vi "Retrieve and visulize data_SE.vi"(10 "stop":bool, 11 "Field/Temperature":i32(slide) min=0 max=36 step=1) -> (0 "X line cut 2":cluster{dbl[], dbl[]}(graph), 1 "slowest":dbl=4.2894631624221803e-07, 2 "2term Intensity":dbl[][](graph), 3 "Intensity Graph":dbl[][](graph), 4 "Y line cut 2":cluster{dbl[], dbl[]}(graph)={[-1.0, -0.95, -0.9, -0.85, -0.8, -0.75, -0.7, -0.65, -0.6, -0.55, -0.5, -0.45, -0.4, -0.35, -0.3, -0.25, -0.2, -0.15, -0.1, -0.05, 0.0, 0.05, 0.1, 0.15, 0.2, 0.25, 0.3, 0.35, 0.4, 0.45, 0.5, 0.55, 0.6, 0.65, 0.7, 0.75, 0.8, 0.85, 0.9, 0.95, 1.0], [0.0, 0.0, 0.0, 0.0, 0.0, 0.0, 0.0, 0.0, 0.0, 0.0, 0.0, 0.0, 0.0, 0.0, 0.0, 0.0, 0.0, 0.0, 0.0, 0.0, 0.0, 0.0, 0.0, 0.0, 0.0, 0.0, 0.0, 0.0, 0.0, 0.0, 0.0, 0.0, 0.0, 0.0, 0.0, 0.0, 0.0, 0.0, 0.0, 0.0, 0.0]})   [LabVIEW 2016]
uses:
  <vilib>/Analysis/3filter.llb/Savitzky-Golay Filter (DBL).vi
  <vilib>/gmath/NI_Gmath.lvlib
  <vilib>/Analysis/NI_AALBase.lvlib
  <vilib>/Analysis/NI_AAL_SigProc.lvlib
panel:
  in  "Voffset - 2T":dbl format="%#_13g"
  out "Vsd vs Vsg":cluster{dbl[], dbl[]}(graph)
  out "Intensity Graph 12":dbl[][](graph)
  in  "file path (use dialog)":path=path "B:/SketchSET/SA03008H.20180718/processed/decimated_21-BG+SG_Sweep+OVERNIGHT"
  out "Scan names 2":string[](array[string])=["DSA_Vsg1", "B", "B"]
  out "Vfast index":dbl=3.0
  out "Vslow index":i32
  out "side points 4Ttemp":i32=8
  out "side points 2Ttemp":i32=12
  in  "side points 4T":i32=8
  in  "side points 2T":i32=12
  in  "Fit Points":dbl=10.0
  in  "T/B     third axis":bool
  in  "color scale":u32[](array[colorbox])=[16711680, 16772608, 6618880, 3381759, 16860, 10420479]
  in  "Voffset -2T":dbl=2e-05 format="%#_6p"
  in  "Voffset-4T":dbl=-5e-05 format="%#_4p"
  in  "Filter retrieved data?":bool=TRUE
  in  "Generate (T) or Visualize (F)":bool
  in  "Tab Control":T1(tab)=enum."3D"
  out "Comments":string="      #Vslow/#Vfast/# of IV curves/BT offset/#discarded IV curves/Manual offset:\n /101/41/1/0/0/0    \n#of fields: 1    \nField period 1 \nDecimate point 10.000000 \nScan names \nDSA_Vsg1\nB\nB \n IGOR\nX// Date: 7/19/2018 7:21 AM\nX// SA03008H\nX// \nX// Source 2 Drain 28 (lockin 1 and 7)\nX// Slow sweeping BG -5 to 5 inc. 0.1V \nX// Fast sweep SG -1 to 1 inc. 0.05V\n\nX// DSA_Vsg1=1.000000\n\nX// \nX// B= 0.000000\n\n\n\n\n\n\n\n\n\n\n\n\n\n\n\n\n\n\n\n\n\n\n\n\n\n\n\n\n\n\n\n\n\n\n\n\n\n\n\n\nX \nX Display/R 'time.SA03008H.20180718.004140'\nX AppendToGraph 'temp.SA03008H.20180718.004140'\nX AppendToGraph 'B.SA03008H.20180718.004140'\nX AppendToGraph 'Vsource.SA03008H.20180718.004140'\nX AppendToGraph 'Lockin0.SA03008H.20180718.004140'\nX AppendToGraph 'Lockin1.SA03008H.20180718.004140'\nX AppendToGraph 'Lockin2.SA03008H.20180718.004140'\nX AppendToGraph 'Lockin3.SA03008H.20180718.004140'\nX AppendToGraph 'Lockin4.SA03008H.20180718.004140'\nX AppendToGraph 'Lockin5.SA03008H.20180718.004140'\nX AppendToGraph 'B_rate.SA03008H.20180718.004140'\nX AppendToGraph 'DC0.SA03008H.20180718.004140'\nX AppendToGraph 'DC1.SA03008H.20180718.004140'\nX AppendToGraph 'DC2.SA03008H.20180718.004140'\nX AppendToGraph 'DC3.SA03008H.20180718.004140'\nX AppendToGraph 'DC4.SA03008H.20180718.004140'\nX AppendToGraph 'DC5.SA03008H.20180718.004140'\nX AppendToGraph 'DC6.SA03008H.20180718.004140'\nX AppendToGraph 'DC7.SA03008H.20180718.004140'\nX Label bottom \"x label\"\nX Label left \"y label\"\nX ModifyGraph rgb('time.SA03008H.20180718.004140')=(65280,0,0)\nX ModifyGraph rgb('temp.SA03008H.20180718.004140')=(65280,18432,0)\nX ModifyGraph rgb('B.SA03008H.20180718.004140')=(65280,36864,0)\nX ModifyGraph rgb('Vsource.SA03008H.20180718.004140')=(65280,55296,0)\nX ModifyGraph rgb('Lockin0.SA03008H.20180718.004140')=(57344,65280,0)\nX ModifyGraph rgb('Lockin1.SA03008H.20180718.004140')=(37376,65280,0)\nX ModifyGraph rgb('Lockin2.SA03008H.20180718.004140')=(18944,65280,0)\nX ModifyGraph rgb('Lockin3.SA03008H.20180718.004140')=(512,65280,0)\nX ModifyGraph rgb('Lockin4.SA03008H.20180718.004140')=(0,65280,17920)\nX ModifyGraph rgb('Lockin5.SA03008H.20180718.004140')=(0,65280,36352)\nX ModifyGraph rgb('B_rate.SA03008H.20180718.004140')=(0,65280,54784)\nX ModifyGraph rgb('DC0.SA03008H.20180718.004140')=(0,57856,65280)\nX ModifyGraph rgb('DC1.SA03008H.20180718.004140')=(0,39424,65280)\nX ModifyGraph rgb('DC2.SA03008H.20180718.004140')=(0,20992,65280)\nX ModifyGraph rgb('DC3.SA03008H.20180718.004140')=(0,2560,65280)\nX ModifyGraph rgb('DC4.SA03008H.20180718.004140')=(17408,0,65280)\nX ModifyGraph rgb('DC5.SA03008H.20180718.004140')=(35840,0,65280)\nX ModifyGraph rgb('DC6.SA03008H.20180718.004140')=(54272,0,65280)\nX ModifyGraph rgb('DC7.SA03008H.20180718.004140')=(65280,0,58368)\nX Legend/C/N=text0/J \"\\\\s('time.SA03008H.20180718.004140') time\\r\\\\s('temp.SA03008H.20180718.004140') temp\\r\\\\s('B.SA03008H.20180718.004140') B\\r\\\\s('Vsource.SA03008H.20180718.004140') Vsource\\r\\\\s('Lockin0.SA03008H.20180718.004140') Lockin0\\r\\\\s('Lockin1.SA03008H.20180718.004140') Lockin1\\r\\\\s('Lockin2.SA03008H.20180718.004140') Lockin2\\r\\\\s('Lockin3.SA03008H.20180718.004140') Lockin3\\r\\\\s('Lockin4.SA03008H.20180718.004140') Lockin4\\r\\\\s('Lockin5.SA03008H.20180718.004140') Lockin5\\r\\\\s('B_rate.SA03008H.20180718.004140') B_rate\\r\\\\s('DC0.SA03008H.20180718.004140') DC0\\r\\\\s('DC1.SA03008H.20180718.004140') DC1\\r\\\\s('DC2.SA03008H.20180718.004140') DC2\\r\\\\s('DC3.SA03008H.20180718.004140') DC3\\r\\\\s('DC4.SA03008H.20180718.004140') DC4\\r\\\\s('DC5.SA03008H.20180718.004140') DC5\\r\\\\s('DC6.SA03008H.20180718.004140') DC6\\r\\\\s('DC7.SA03008H.20180718.004140') DC7\"\nX ModifyGraph mirror(bottom)=1\nX ModifyGraph width=216\nX ModifyGraph height={Aspect,0.6}\nX ModifyGraph Log(bottom)=0\nX ModifyGraph Log(left)=0\nX \n"
  in  "Additional comments":string
  in  "Field Period":i32=1
  in  "# of fields/Temperatures":i32=1
  in  "File or Folder Path":path=path "B:/SketchSET/SA03008H.20180718/21-BG+SG_Sweep+OVERNIGHT"
  in  "Processed data folder":path=path "B:/SketchSET/SA03008H.20180718/processed"
  in  "IV file name":string="decimated_21-BG+SG_Sweep+OVERNIGHT"
  in  "IV setup":T2={"# of Vslow"=101, "# Vfast"=41, "#IV Curves at each gate"=1, "B/T offset"=0, "Discard first # curves"=0, "Manual offset"=0}
  in  "Scan names":string[](array[string])=["DSA_Vsg1", "B", "B"]
  in  "Portion of data":cluster{dbl, dbl}(slide)={1.0, 0.0} scale=0.0..1.0
  in  "Decimate point":dbl=10.0 format="%#_1f"
  in  "Extract parameters from comments?":bool=TRUE
  in  "index 2":T3={"A"=3, "B"=5, "C"=3, "D"=5, "E"=3, "N1"=2, "N2"=2, "N3"=3, "N4"=4, "A 1"=3, "A 2"=3, "C 1"=3, "C 2"=3, "E 2"=4}
  out "dV/dI 2T":cluster{dbl[], dbl[]}[](graph)
  out "dV/dI vs I":cluster{dbl[], dbl[]}[](graph)
  out "IV 2T":cluster{dbl[], dbl[]}[](graph)
  out "dI/dV 2T":cluster{dbl[], dbl[]}[](graph)
  out "dI/dV vs V":cluster{dbl[], dbl[]}[](graph)
  out "IV":cluster{dbl[], dbl[]}[](graph)
  out "IV slow 2T":cluster{dbl[], dbl[]}[](graph)
  out "dI/dV slow 2T":cluster{dbl[], dbl[]}[](graph)
  out "IV slow 4T":cluster{dbl[], dbl[]}[](graph)
  out "dI/dV slow 4T":cluster{dbl[], dbl[]}[](graph)
  out "IV vary 3rd 2T":cluster{dbl[], dbl[]}[](graph)
  out "dI/dV vary 3rd 2T":cluster{dbl[], dbl[]}[](graph)
  out "IV vary 3rd 4T":cluster{dbl[], dbl[]}[](graph)
  out "dI/dV vary 3rd 4T":cluster{dbl[], dbl[]}[](graph)
  out "Intensity Graph 2":dbl[][](graph)
  in  "X Low":dbl=-0.1 format="%#_6p"
  in  "X High":dbl=0.1 format="%#_6p"
  in  "X Step":dbl=5e-05 format="%#_6p"
  in  "Log scale?":bool
  in  "Log scale?":bool
  in  "No scale?":bool
  in  "Breakdown Low":dbl=-0.1 format="%#_6p"
  in  "Breakdown High":dbl=0.2 format="%#_6p"
  out "X scale":cluster{dbl, "X Step":dbl}={-0.09995000000000001, "X Step"=5e-05}
  out "Y scale":cluster{"Real Voltage":dbl, dbl}={"Real Voltage"=-1.0, 0.050000000000000044}
  in  "fake point value":dbl format="%#_6p"
  out "Transconductance":dbl[][](graph)
  in  "derivative bin size":dbl=15.0
  out "Field":dbl=-3.687258687258687
  out "X line cut 3":cluster{dbl[], dbl[]}(graph)
  out "X line cut 7":cluster{dbl[], dbl[]}(graph)={array[399 elements], [-0.0, -0.0, -0.0, -0.0, -0.0, -0.0, -0.0, -0.0, -0.0, -0.0, -0.0, -0.0, -0.0, -0.0, -0.0, -0.0, -0.0, -0.0, -0.0, -0.0, -0.0, -0.0, -0.0, -0.0, -0.0, -0.0, -0.0, -0.0, -0.0, -0.0, -0.0, -0.0, -0.0, -0.0, -0.0, -0.0, -0.0, -0.0, -0.0, -0.0, -0.0, -0.0, -0.0, -0.0, -0.0, -0.0, -0.0, -0.0, -0.0, -0.0, -0.0, -0.0, -0.0, -0.0, -0.0, -0.0, -0.0, -0.0, -0.0, -0.0, -0.0, -0.0, -0.0, -0.0, -0.0, -0.0, -0.0, -0.0, -0.0, -0.0, -0.0, -0.0, -0.0, -0.0, -0.0, -0.0, -0.0, -0.0, -0.0, -0.0, -0.0, -0.0, -0.0, -0.0, -0.0, -0.0, -0.0, -0.0, -0.0, -0.0, -0.0, -0.0, -0.0, -0.0, -0.0, -0.0, -0.0, -0.0, -0.0, -0.0, -0.0, -0.0, -0.0, -0.0, -0.0, -0.0, -0.0, -0.0, -0.0, -0.0, -0.0, -0.0, -0.0, -0.0, -0.0, -0.0, -0.0, -0.0, -0.0, -0.0, -0.0, -0.0, -0.0, -0.0, -0.0, -0.0, -0.0, -0.0, -0.0, -0.0, -0.0, -0.0, -0.0, -0.0, -0.0, -0.0, -0.0, -0.0, -0.0, -0.0, -0.0, -0.0, -0.0, -0.0, -0.0, -0.0, -0.0, -0.0, -0.0, -0.0, -0.0, -0.0, -0.0, -0.0, -0.0, -0.0, -0.0, -0.0, -0.0, -0.0, -0.0, -0.0, -0.0, -0.0, -0.0, -0.0, -0.0, -0.0, -0.0, -0.0, -0.0, -0.0, -0.0, -0.0, -0.0, -0.0, -0.0, -0.0, -0.0, -0.0, -0.0, -0.0, -0.0, -0.0, -0.0, -0.0, -0.0, -0.0, -0.0, -0.0, -0.0, -0.0, -0.0, -0.0, -0.0, -0.0, -0.0, -0.0, -0.0, -0.0, -0.0, -0.0, -0.0, -0.0, -0.0, -0.0, -0.0, -0.0, -0.0, -0.0, -0.0, -0.0, -0.0, -0.0, -0.0, -0.0, -0.0, -0.0, -0.0, -0.0, -0.0, -0.0, -0.0, -0.0, -0.0, -0.0, -0.0, -0.0, -0.0, -0.0, -0.0, -0.0, -0.0, -0.0, -0.0, -0.0, -0.0, -0.0, -0.0, -0.0, -0.0, -0.0, -0.0, -0.0, -0.0, -0.0, -0.0, -0.0, -0.0, -0.0, -0.0, -0.0, -0.0, -0.0, -0.0, -0.0, -0.0, -0.0, -0.0, -0.0, -0.0, -0.0, -0.0, -0.0, -0.0, -0.0, -0.0, -0.0, -0.0, -0.0, -0.0, -0.0, -0.0, -0.0, -0.0, -0.0, -0.0, -0.0, -0.0, -0.0, -0.0, -0.0, -0.0, -0.0, -0.0, -0.0, -0.0, -0.0, -0.0, -0.0, -0.0, -0.0, -0.0, -0.0, -0.0, -0.0, -0.0, -0.0, -0.0, -0.0, -0.0, -0.0, -0.0, -0.0, -0.0, -0.0, -0.0, -0.0, -0.0, -0.0, -0.0, -0.0, -0.0, -0.0, -0.0, -0.0, -0.0, -0.0, -0.0, -0.0, -0.0, -0.0, -0.0, -0.0, -0.0, -0.0, -0.0, -0.0, -0.0, -0.0, -0.0, -0.0, -0.0, -0.0, -0.0, -0.0, -0.0, -0.0, -0.0, -0.0, -0.0, -0.0, -0.0, -0.0, -0.0, -0.0, -0.0, -0.0, -0.0, -0.0, -0.0, -0.0, -0.0, -0.0, -0.0, -0.0, -0.0, -0.0, -0.0, -0.0, -0.0, -0.0, -0.0, -0.0, -0.0, -0.0, -0.0, -0.0, -0.0, -0.0, -0.0, -0.0, -0.0, -0.0, -0.0, -0.0, -0.0, -0.0, -0.0, -0.0, -0.0, -0.0, -0.0, -0.0, -0.0, -0.0, -0.0, -0.0, -0.0, -0.0, -0.0, -0.0, -0.0, -0.0, -0.0, -0.0, -0.0, -0.0, -0.0]}
  out "Y line cut 8":cluster{dbl[], dbl[]}(graph)={[-1.0, -0.95, -0.9, -0.85, -0.8, -0.75, -0.7, -0.65, -0.6, -0.55, -0.5, -0.45, -0.4, -0.35, -0.3, -0.25, -0.2, -0.15, -0.1, -0.05, 0.0, 0.05, 0.1, 0.15, 0.2, 0.25, 0.3, 0.35, 0.4, 0.45, 0.5, 0.55, 0.6, 0.65, 0.7, 0.75, 0.8, 0.85, 0.9, 0.95, 1.0], [-0.0, -0.0, -0.0, -0.0, -0.0, -0.0, -0.0, -0.0, -0.0, -0.0, -0.0, -0.0, -0.0, -0.0, -0.0, -0.0, -0.0, -0.0, -0.0, -0.0, -0.0, -0.0, -0.0, -0.0, -0.0, -0.0, -0.0]}
  out "Y line cut":cluster{"Vfast":dbl[], dbl[]}(graph)
  out "X line cut":cluster{dbl[], dbl[]}(graph)
  out "2 term trans":dbl[][](graph)
  in  "X Step 2T":dbl=4e-05 format="%#_6p"
  in  "X High 2T":dbl=0.1 format="%#_6p"
  in  "X Low 2T":dbl=-0.1 format="%#_6p"
  in  "Log scale?":bool
  in  "Log scale?":bool
  in  "fake point value 2":dbl format="%#_6p"
  out "2term trans X line cut":cluster{dbl[], dbl[]}(graph)
  out "2term trans Y line cut":cluster{"Vfast":dbl[], dbl[]}(graph)
  in  "e^2/h?":bool
  out "2term Intensity Current vs. Voltage":dbl[][](graph)
  in  "width X 6":dbl=1e-09 min=1.0 format="%#_6p"
  in  "width Y 6":dbl=1e-09 min=1.0 format="%#_6p"
  out "Y line cut 6":cluster{"Vfast":dbl[], dbl[]}(graph)={"Vfast"=[-5.0, -4.9, -4.8, -4.7, -4.6, -4.5, -4.4, -4.3, -4.2, -4.1, -4.0, -3.9, -3.8, -3.7, -3.5999999999999996, -3.5, -3.4, -3.3, -3.2, -3.0999999999999996, -3.0, -2.9, -2.8, -2.6999999999999997, -2.5999999999999996, -2.5, -2.4, -2.3, -2.1999999999999997, -2.0999999999999996, -2.0, -1.9, -1.7999999999999998, -1.6999999999999997, -1.5999999999999996, -1.5, -1.4, -1.2999999999999998, -1.1999999999999997, -1.0999999999999996, -1.0, -0.8999999999999995, -0.7999999999999998, -0.7000000000000002, -0.5999999999999996, -0.5, -0.39999999999999947, -0.2999999999999998, -0.1999999999999993, -0.09999999999999964, 0.0, 0.10000000000000053, 0.20000000000000018, 0.3000000000000007, 0.40000000000000036, 0.5, 0.6000000000000005, 0.7000000000000002, 0.8000000000000007, 0.9000000000000004, 1.0, 1.1000000000000005, 1.2000000000000002, 1.3000000000000007, 1.4000000000000004, 1.5, 1.6000000000000005, 1.7000000000000002, 1.8000000000000007, 1.9000000000000004, 2.0, 2.1000000000000005, 2.2, 2.3000000000000007, 2.4000000000000004, 2.5, 2.6000000000000005, 2.7, 2.8000000000000007, 2.9000000000000004, 3.0, 3.0999999999999996, 3.200000000000001, 3.3000000000000007, 3.4000000000000004, 3.5, 3.5999999999999996, 3.700000000000001, 3.8000000000000007, 3.9000000000000004, 4.0, 4.1, 4.200000000000001, 4.300000000000001, 4.4, 4.5, 4.600000000000001, 4.700000000000001, 4.800000000000001, 4.9, 5.0], [0.02727272727272727, 0.02727272727272727, 0.02727272727272727, 0.02727272727272727, 0.02727272727272727, 0.02727272727272727, 0.02727272727272727, 0.02727272727272727, 0.02727272727272727, 0.02727272727272727, 0.02727272727272727, 0.02727272727272727, 0.02727272727272727, 0.02727272727272727, 0.02727272727272727, 0.02727272727272727, 0.02727272727272727, 0.02727272727272727, 0.02727272727272727, 0.02727272727272727, 0.02727272727272727, 0.02727272727272727, 0.02727272727272727, 0.02727272727272727, 0.02727272727272727, 0.02727272727272727, 0.02727272727272727, 0.02727272727272727, 0.02727272727272727, 0.02727272727272727, 0.02727272727272727, 0.02727272727272727, 0.02727272727272727, 0.02727272727272727, 0.02727272727272727, 0.02727272727272727, 0.02727272727272727, 0.02727272727272727, 0.02727272727272727, 0.02727272727272727, 0.02727272727272727, 0.02727272727272727, 0.02727272727272727, 0.02727272727272727, 0.02727272727272727, 0.02727272727272727, 0.02727272727272727, 0.02727272727272727, 0.02727272727272727, 0.02727272727272727, 0.02727272727272727, 0.02727272727272727, 0.02727272727272727, 0.02727272727272727, 0.02727272727272727, 0.02727272727272727, 0.02727272727272727, 0.02727272727272727, 0.02727272727272727, 0.02727272727272727, 0.02727272727272727, 0.02727272727272727, 0.02727272727272727, 0.02727272727272727, 0.02727272727272727, 0.02727272727272727, 0.02727272727272727, 0.02727272727272727, 0.02727272727272727, 0.02727272727272727, 0.02727272727272727, 0.02727272727272727, 0.02727272727272727, 0.02727272727272727, 0.02727272727272727, 0.02727272727272727, 0.02727272727272727, 0.02727272727272727, 0.02727272727272727, 0.02727272727272727, 0.02727272727272727, 0.02727272727272727, 0.02727272727272727, 0.02727272727272727, 0.02727272727272727, 0.02727272727272727, 0.02727272727272727, 0.02727272727272727, 0.02727272727272727, 0.02727272727272727, 0.02727272727272727, 0.02727272727272727, 0.02727272727272727, 0.02727272727272727, 0.02727272727272727, 0.02727272727272727, 0.02727272727272727, 0.02727272727272727, 0.02727272727272727, 0.02727272727272727, 0.02727272727272727]}
  out "X line cut 6":cluster{dbl[], dbl[]}(graph)
  out "Y line cut 5":cluster{"Vfast":dbl[], dbl[]}(graph)={"Vfast"=[-1.0, -0.95, -0.9, -0.85, -0.8, -0.75, -0.7, -0.65, -0.6, -0.55, -0.5, -0.45, -0.4, -0.35, -0.3, -0.25, -0.2, -0.15, -0.1, -0.05, 0.0, 0.05, 0.1, 0.15, 0.2, 0.25, 0.3, 0.35, 0.4, 0.45, 0.5, 0.55, 0.6, 0.65, 0.7, 0.75, 0.8, 0.85, 0.9, 0.95, 1.0], [0.049999999999999996, 0.049999999999999996, 0.049999999999999996, 0.049999999999999996, 0.049999999999999996, 0.049999999999999996, 0.049999999999999996, 0.049999999999999996, 0.049999999999999996, 0.049999999999999996, 0.049999999999999996, 0.049999999999999996, 0.049999999999999996, 0.049999999999999996, 0.049999999999999996, 0.049999999999999996, 0.049999999999999996, 0.049999999999999996, 0.049999999999999996, 0.049999999999999996, 0.049999999999999996, 0.049999999999999996, 0.049999999999999996, 0.049999999999999996, 0.049999999999999996, 0.049999999999999996, 0.049999999999999996, 0.049999999999999996, 0.049999999999999996, 0.049999999999999996, 0.049999999999999996, 0.049999999999999996, 0.049999999999999996, 0.049999999999999996, 0.049999999999999996, 0.049999999999999996, 0.049999999999999996, 0.049999999999999996, 0.049999999999999996, 0.049999999999999996, 0.049999999999999996]}
  out "X line cut 5":cluster{dbl[], dbl[]}(graph)
  out "Intensity Graph 6":dbl[][](graph)
  in  "X Step 4t":dbl=1e-10 format="%#_6p"
  in  "X High 4t":dbl=3e-08 format="%#_6p"
  in  "X Low 4t":dbl=-3e-08 format="%#_6p"
  in  "Log scale? 3":bool
  in  "Log scale? 2":bool
  out "Intensity Graph 5":dbl[][](graph)
  in  "fake point value 3":dbl=0.05 format="%#_6p"
  in  "width X 5":dbl=1e-09 min=1.0 format="%#_6p"
  in  "width Y 5":dbl=1e-09 min=1.0 format="%#_6p"
  out "Y line cut 4":cluster{"Vfast":dbl[], dbl[]}(graph)
  out "X line cut 4":cluster{dbl[], dbl[]}(graph)
  out "Intensity Graph 8":dbl[][](graph)
  in  "X Step 2t":dbl=1e-11 format="%#_6p"
  in  "X High 2t":dbl=1e-09 format="%#_6p"
  in  "X Low 2t":dbl=-2e-09 format="%#_6p"
  in  "Log scale? 5":bool
  in  "Log scale? 4":bool
  out "Intensity Graph 7":dbl[][](graph)
  in  "fake pt value 4":dbl=0.05 format="%#_6p"
  out "Intensity Graph 11":dbl[][](graph)
  out "Intensity Graph 10":dbl[][](graph)
  out "Intensity Graph 9":dbl[][](graph)
  out "Transconductance 2":dbl[][](graph)
  in  "derivative bin size 2":dbl=10.0
  in  "width":i32=3 min=3
  in  "threshold":dbl format="%0.2f"
  out "vertical peak diff":dbl[](array[numeric])
  out "Array 2":dbl[](array[numeric])
  out "Y line cut 9":cluster{dbl[], dbl[]}[](graph)
  in  "width 2":i32=3 min=3
  in  "threshold 2":dbl format="%0.2f"
  in  "calc alpha?":bool
  out "XY Graph":cluster{dbl[], dbl[]}(graph)
  # "I+"
  # "V+"
  # "Vsg1"
  # "Vsgw"
  # "Vsg2"
  # "V-"
  # "I-"
  # "Output"
  # "Vfast"
  # "Vslow"
  # "Vslowest"
  # "Vfast"
  # "Vslow"
  # "Vslowest"
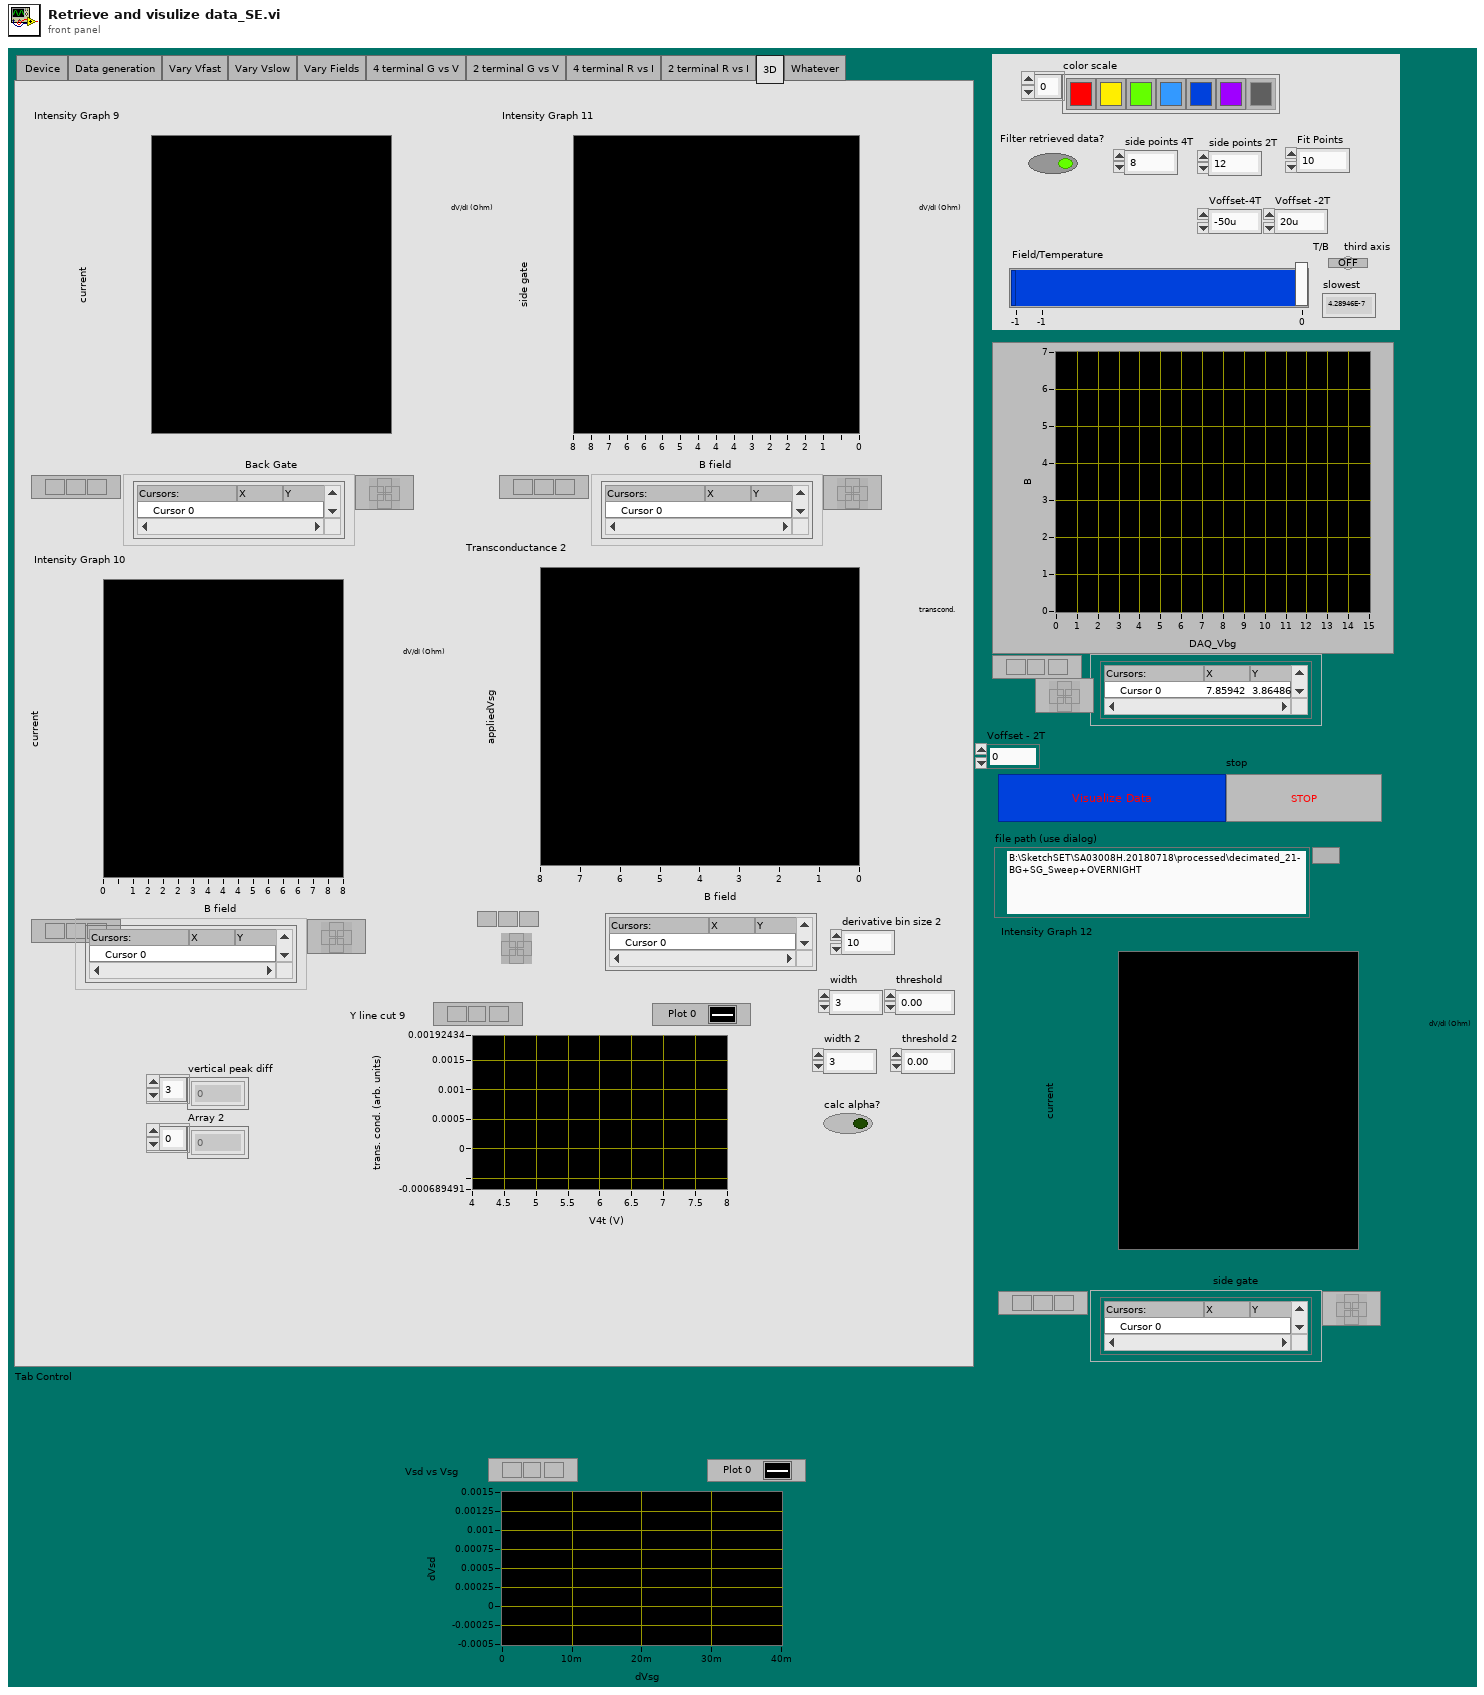
[diagram p1: front panel]
types:
  T1 = enum32{"Device ", "Data generation", "Vary Vfast", "Vary Vslow", "Vary Fields", "4 terminal G vs V", "2 terminal G vs V", "4 terminal R vs I", "2 terminal R vs I", "3D", "Whatever"}
  T2 = cluster{"# of Vslow":i32, "# Vfast":i32, "#IV Curves at each gate":i32, "B/T offset":i32, "Discard first # curves":i32, "Manual offset":i32}
  T3 = cluster{"A":i32, "B":i32, "C":i32, "D":i32, "E":i32, "N1":i32, "N2":i32, "N3":i32, "N4":i32, "A 1":i32, "A 2":i32, "C 1":i32, "C 2":i32, "E 2":i32}
  T4 = enum16{"open", "replace", "create", "open or create", "replace or create", "replace or create with confirmation"}
  T5 = cluster{"IV":cluster{dbl[], dbl[]}[][][], "IV-2T":cluster{dbl[], dbl[]}[][][], "Vfast":dbl[][], "Vslow":dbl[], "Vslowest":dbl[], "Comments":string, "Scan names":string[]}[]
  T6 = cluster{"IV":cluster{dbl[], dbl[]}[][][], "IV-2T":cluster{dbl[], dbl[]}[][][], "Vfast":dbl[][], "Vslow":dbl[], "Vslowest":dbl[], "Comments":string, "Scan names":string[]}
  T7 = cluster{"Decimated Array":dbl[], "Decimated Array":dbl[]}
  T8 = cluster{"Decimated Array":dbl[], "Decimated Array":dbl[]}[][][]
  T9 = cluster{"Decimated Array":dbl[], "Filtered X":dbl[]}
  T10 = cluster{"Decimated Array":dbl[], "Decimated Array":dbl[]}[][]
  T11 = cluster{"Decimated Array":dbl[], "Decimated Array":dbl[]}[]
  T12 = cluster{"X Low 2T":dbl, "X High 2T":dbl, "X Step 2T":dbl, "Voffset -2T":dbl}
  T13 = cluster{"Decimated X values":dbl[], "Transconductance":dbl[]}
  T14 = cluster{"X Low 2t":dbl, "X High 2t":dbl, "X Step 2t":dbl, "Voffset - 2T":dbl}
  T15 = cluster{"IV":cluster{dbl[], dbl[]}[][][], "IV-2T":cluster{dbl[], dbl[]}[][][], "Vfast":dbl[][], "Vslow":dbl[], dbl[], string, "Scan names":string[]}
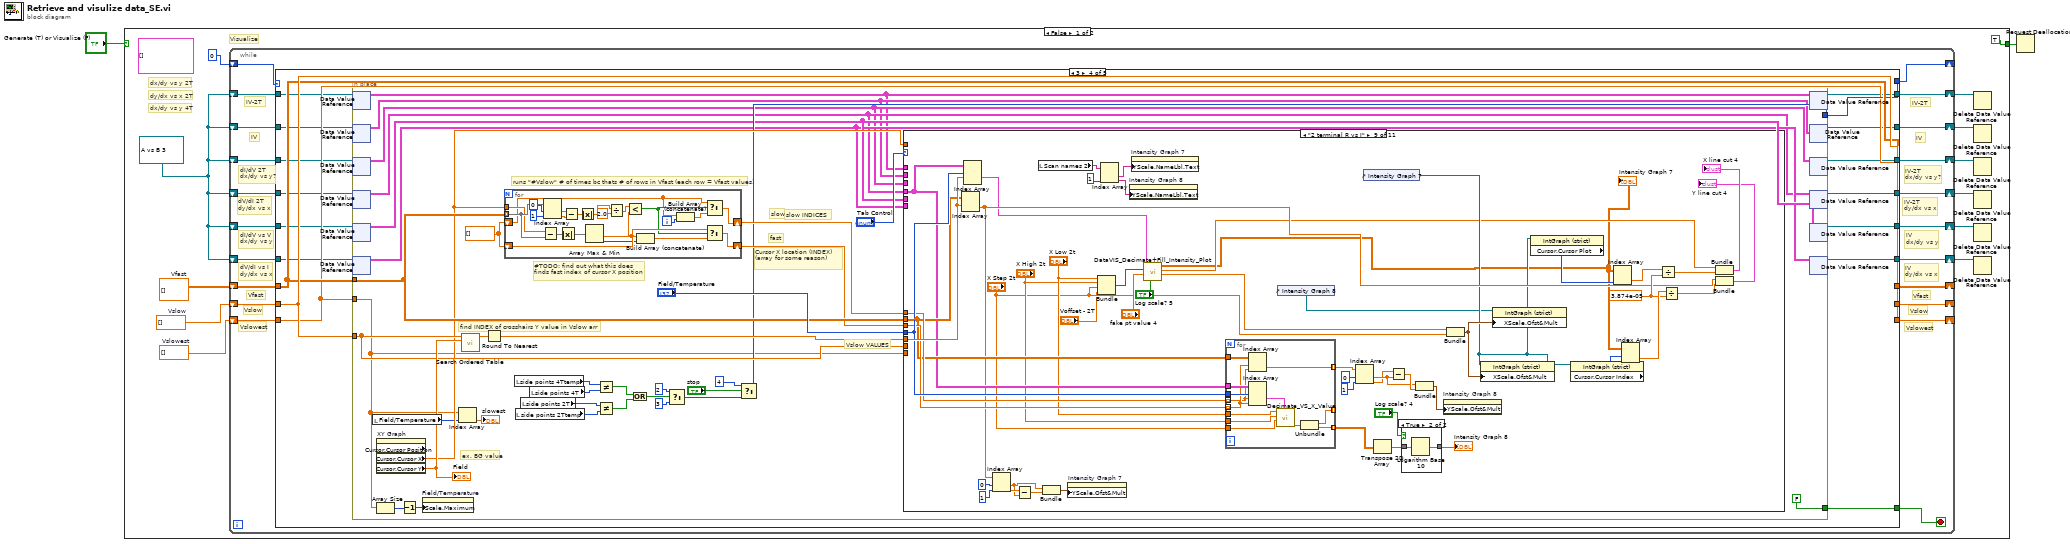
[diagram p0: block diagram]
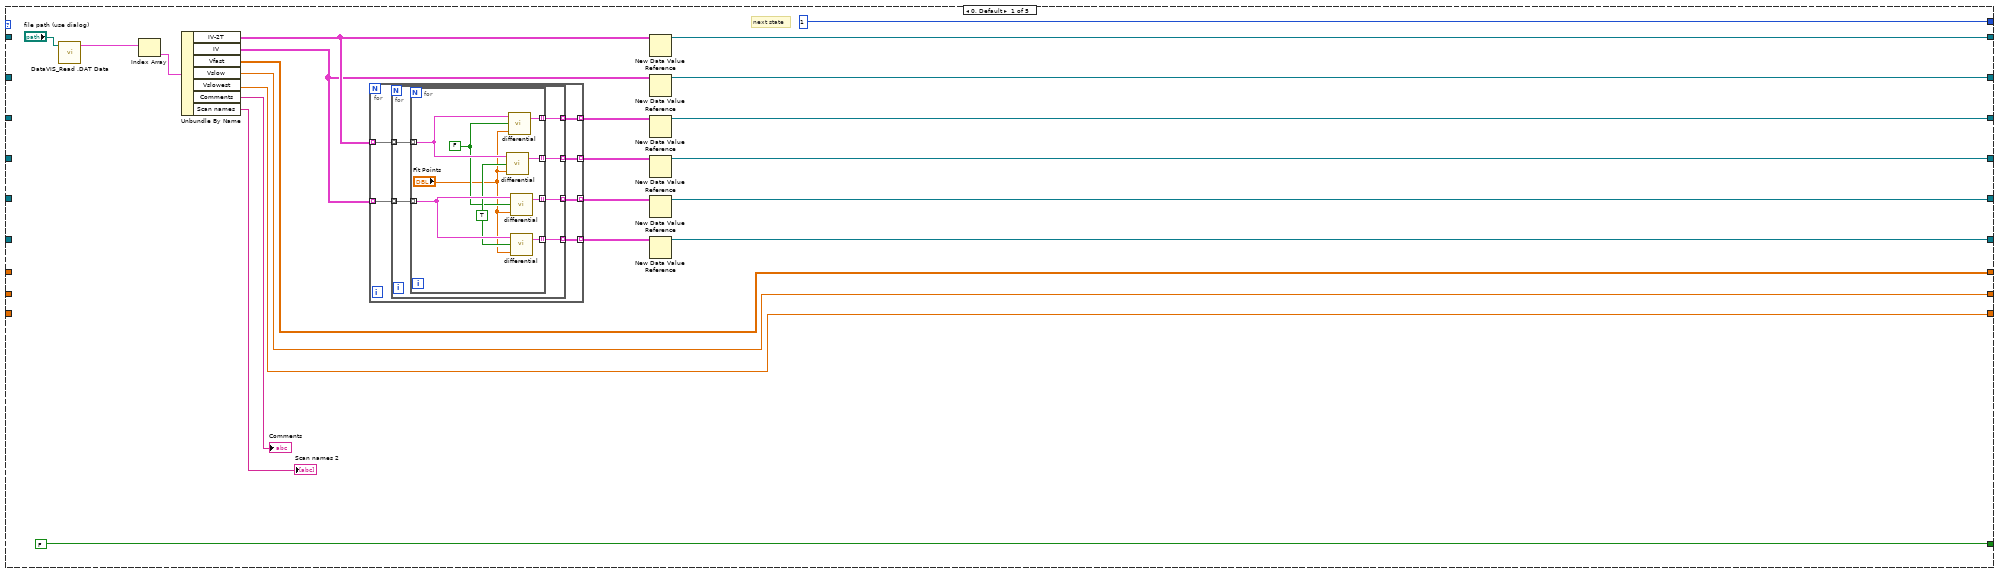
[diagram p2: hidden frame]
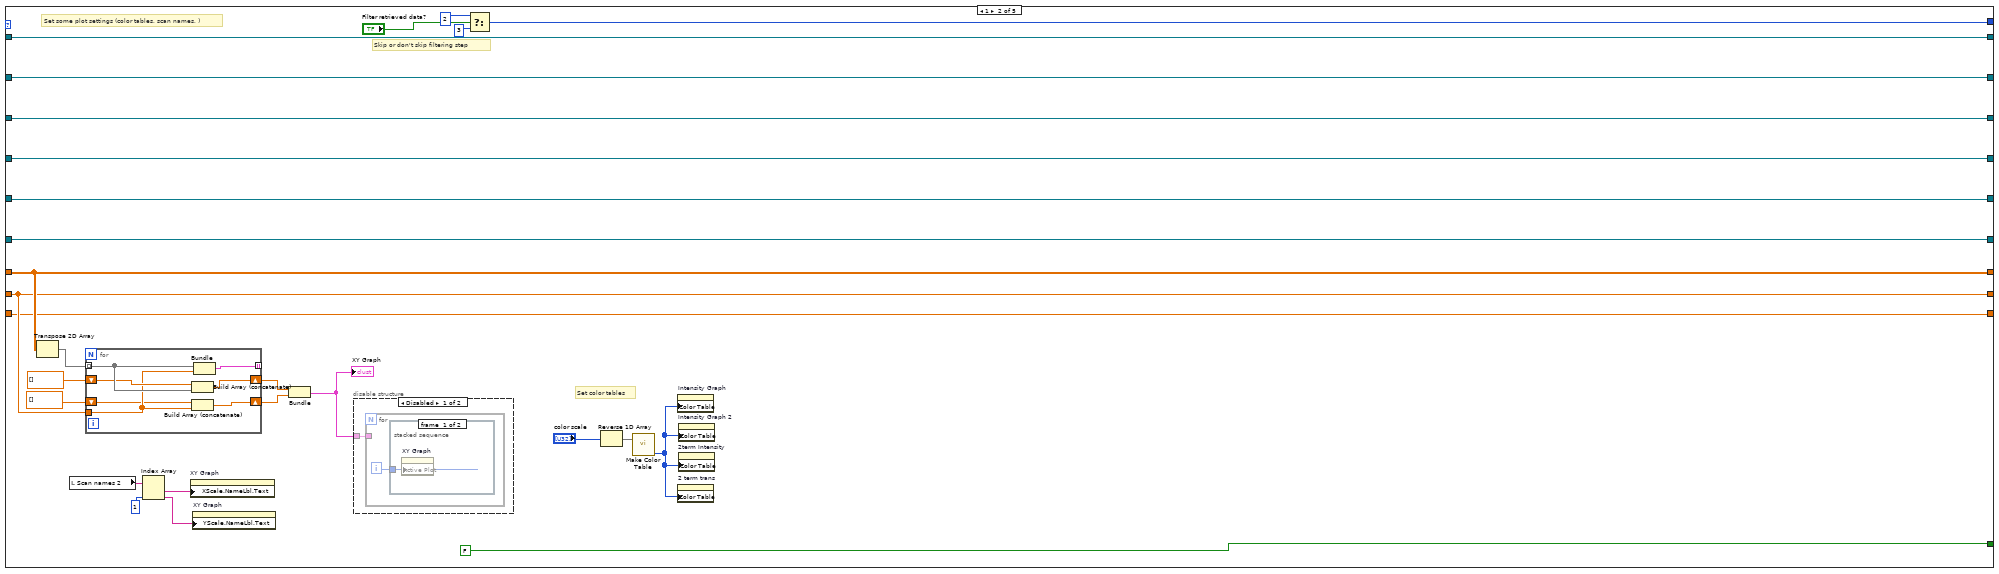
[diagram p3: hidden frame]
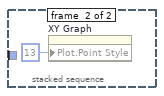
[diagram p4: hidden frame]
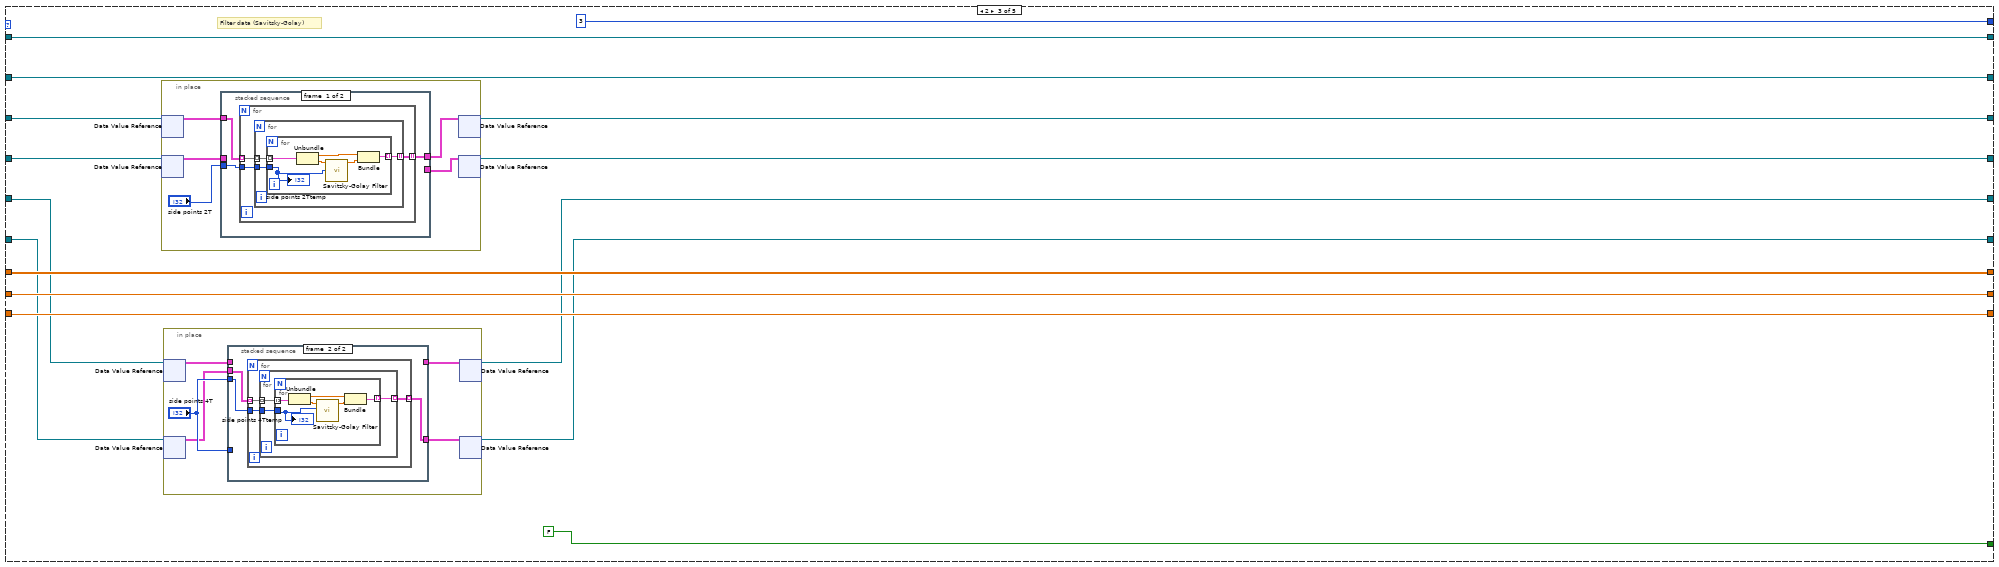
[diagram p6: hidden frame]
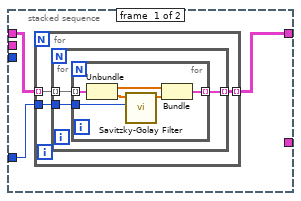
[diagram p7: hidden frame]
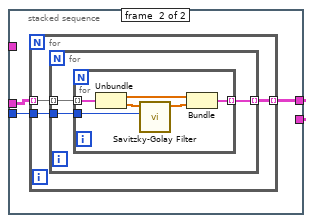
[diagram p8: hidden frame]
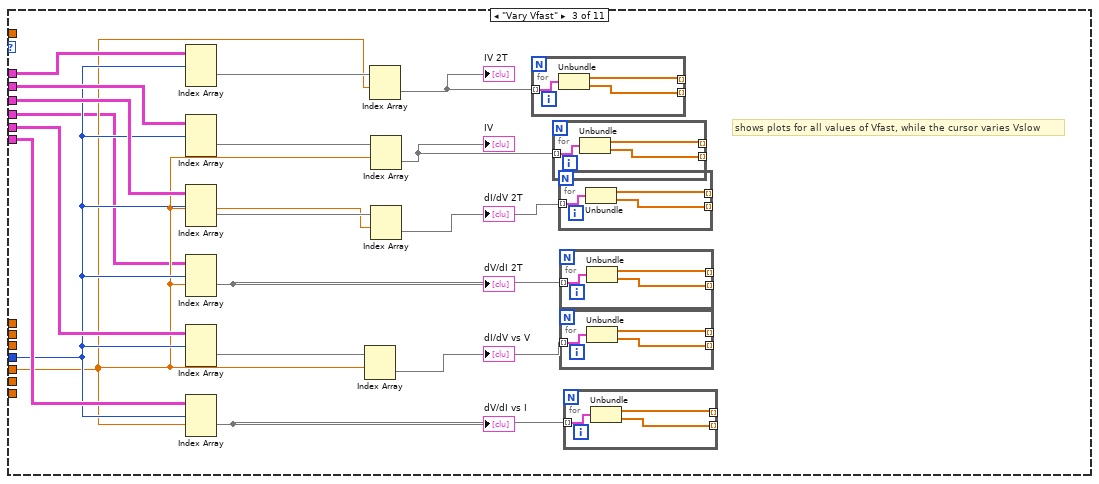
[diagram p11: hidden frame]
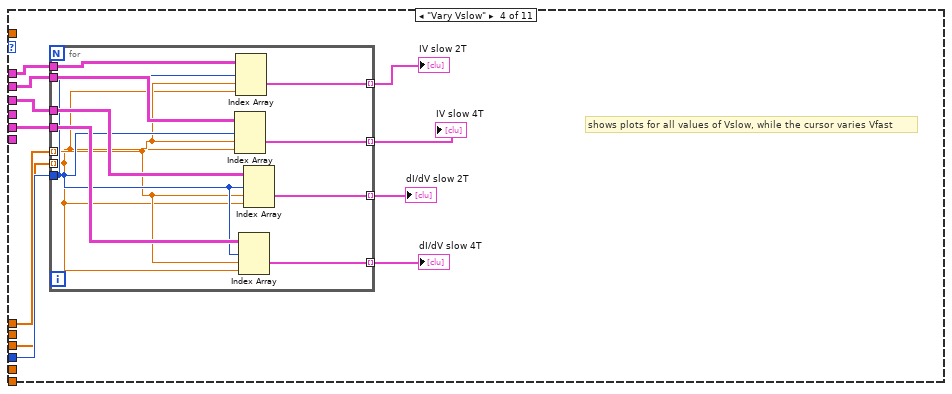
[diagram p12: hidden frame]
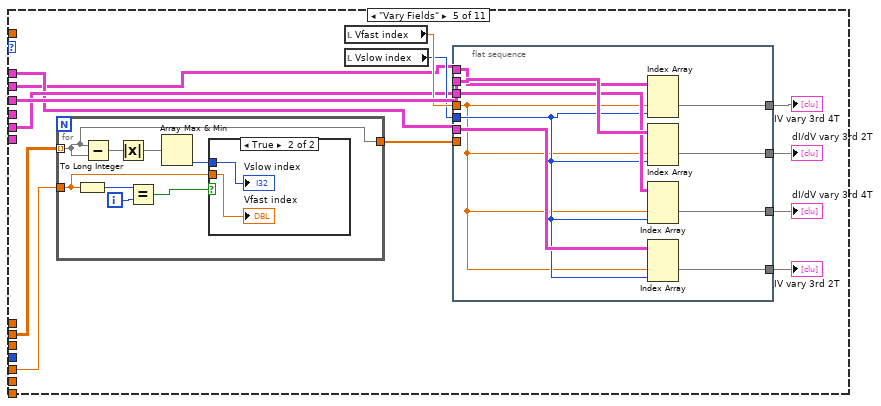
[diagram p13: hidden frame]
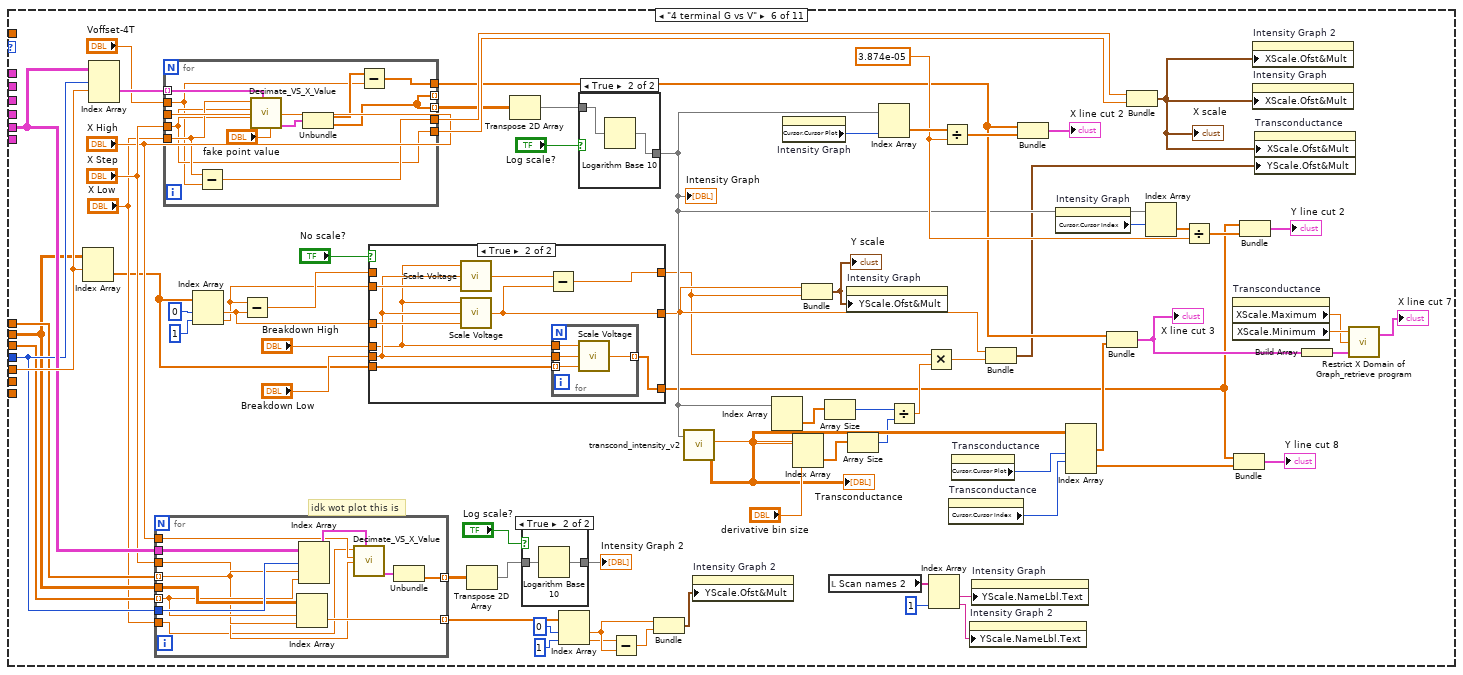
[diagram p15: hidden frame]
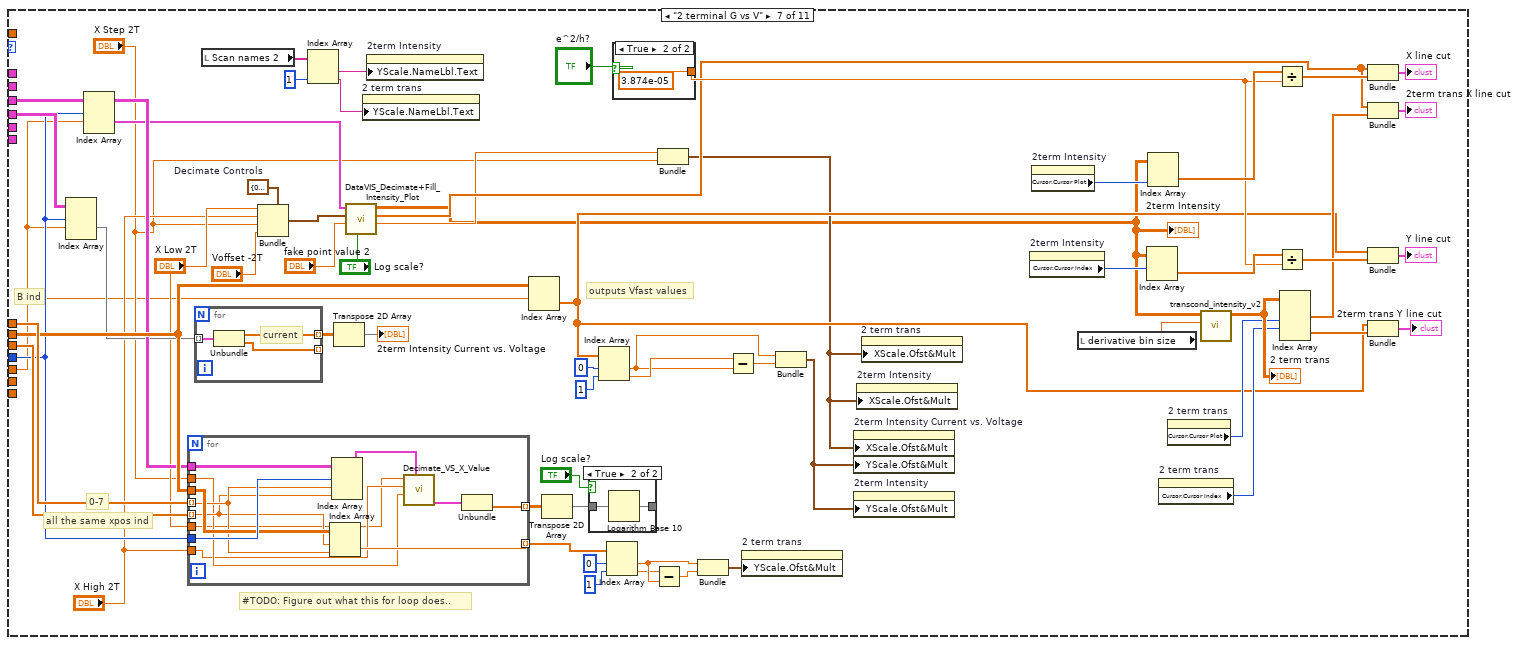
[diagram p19: hidden frame]
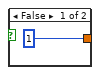
[diagram p20: hidden frame]
diagram:
  n1 = case shown="False" "Generate (T) or Visualize (F)" {
    tunnel: [TRUE TRUE] -> w1
    frame False {
      w3 = dbl[] []  # Vslowest
      w11 = refnum<data-value> refnum ("data value reference")
      w13 = dbl[] []  # Vslow
      w14 = dbl[][] []  # Vfast
      (unwired) cluster{dbl[], dbl[]}[][][] [] ("IV")
      # "Visualize"
      # "dx/dy vs y 4T"
      # "dy/dx vs x 2T"
      # "dx/dy vs y 2T"
      n2 = while {
        shift-right: [w31] -> _
        shift-left: 0 -> [w35]
        shift-right: [w15] -> w10
        shift-left: w11 -> [w16]
        shift-right: [w26] -> w9
        shift-left: w11 -> [w21]
        shift-right: [w25] -> w8
        shift-left: w11 -> [w20]
        shift-right: [w24] -> w7
        shift-left: w11 -> [w19]
        shift-right: [w23] -> w6
        shift-left: w11 -> [w18]
        shift-right: [w22] -> w5
        shift-left: w11 -> [w17]
        shift-right: [w34] -> _
        shift-left: w14 -> [w30]
        shift-right: [w33] -> _
        shift-left: w13 -> [w29]
        shift-right: [w32] -> _
        shift-left: w3 -> [w28]
        stop <- w27 stop-if-true
        # "dI/dV vs V\ndx/dy vs y"
        # "dV/dI vs I\ndy/dx vs x"
        # "dV/dI 2T\ndy/dx vs x"
        # "dI/dV 2T\ndx/dy vs y?"
        # "IV"
        # "IV-2T"
        # "Vfast"
        # "Vslowest"
        # "Vslow"
        # "IV\ndx/dy vs y"
        # "IV\ndy/dx vs x"
        # "IV-2T\ndy/dx vs x"
        # "IV-2T\ndx/dy vs y?"
        # "IV"
        # "IV-2T"
        # "Vfast"
        # "Vslowest"
        # "Vslow"
        n3 = case shown="3" w35 {
          tunnel: [w54 w104 w122 w206 w848] -> w26
          tunnel: [w52 w103 w118 w204 w846] -> w24
          tunnel: [w51 w98 w131 w203 w845] -> w23
          tunnel: [w50 w99 w130 w202 w844] -> w22
          tunnel: [w37 w102 w128 w217 w850] -> w34
          tunnel: [w36 w101 w127 w218 w854] -> w33
          tunnel: [w57 w100 w126 w214 w853] -> w32
          tunnel: w16 -> [_ w79 w124 w213 w849]
          tunnel: w20 -> [_ w80 w121 w210 w847]
          tunnel: w21 -> [_ w104 w123 w211 w848]
          tunnel: w19 -> [_ w103 w120 w209 w846]
          tunnel: w18 -> [_ w98 w131 w208 w845]
          tunnel: w17 -> [_ w99 w130 w207 w844]
          tunnel: [1 w91 3 w216 4] -> w31
          tunnel: w30 -> [_ w102 w128 w217 w850]
          tunnel: w29 -> [_ w101 w127 w218 w854]
          tunnel: w28 -> [_ w100 w126 w214 w853]
          tunnel: [FALSE FALSE FALSE w215 TRUE] -> w27
          tunnel: [w53 w80 w119 w205 w847] -> w25
          tunnel: [w49 w79 w117 w212 w849] -> w15
          frame 0, Default {
            # "next state"
            n4 = call "DataVIS_Read .DAT Data.vi"("file path (use dialog)"="file path (use dialog)") -> ("Array"=w48:T5)  [unwired: 9 in, 1 out]
            n5 = Index Array(array=w48) -> (element=w47:T6)  [unwired: 1 in]
            n6 = Unbundle By Name(w47) -> ("IV-2T"=w39:cluster{dbl[], dbl[]}[][][], "IV"=w38:cluster{dbl[], dbl[]}[][][], "Vfast"=w37:dbl[][], "Vslow"=w36:dbl[], "Vslowest"=w57:dbl[], "Comments"=→"Comments":string, "Scan names"=→"Scan names 2":string[])
            n7 = for {
              tunnel: w38 -> [w63] mode=indexing
              tunnel: [w62] -> w40 mode=indexing
              tunnel: [w61] -> w41 mode=indexing
              tunnel: w39 -> [w60] mode=indexing
              tunnel: [w59] -> w42 mode=indexing
              tunnel: [w58] -> w43 mode=indexing
              n8 = for {
                tunnel: w63 -> [w69] mode=indexing
                tunnel: [w68] -> w62 mode=indexing
                tunnel: [w67] -> w61 mode=indexing
                tunnel: w60 -> [w66] mode=indexing
                tunnel: [w65] -> w59 mode=indexing
                tunnel: [w64] -> w58 mode=indexing
                n9 = for {
                  tunnel: w69 -> [w77] mode=indexing
                  tunnel: [w78] -> w68 mode=indexing
                  tunnel: [w75] -> w67 mode=indexing
                  tunnel: w66 -> [w74] mode=indexing
                  tunnel: [w71] -> w65 mode=indexing
                  tunnel: [w70] -> w64 mode=indexing
                  w73 = FALSE ("dy/dx vs x")
                  w76 = TRUE ("dy/dx vs x")
                  n10 = call <userlib>:"differential.vi"("Numeric"="Fit Points", "dy/dx vs x"=w76, "A vs B 2"=w74) -> ("A vs B 3"=w71:T7)  [unwired: 1 in]
                  n11 = call <userlib>:"differential.vi"("Numeric"="Fit Points", "dy/dx vs x"=w73, "A vs B 2"=w74) -> ("A vs B 3"=w70:T7)  [unwired: 1 in]
                  n12 = call <userlib>:"differential.vi"("Numeric"="Fit Points", "dy/dx vs x"=w73, "A vs B 2"=w77) -> ("A vs B 3"=w75:T7)  [unwired: 1 in]
                  n13 = call <userlib>:"differential.vi"("Numeric"="Fit Points", "dy/dx vs x"=w76, "A vs B 2"=w77) -> ("A vs B 3"=w78:T7)  [unwired: 1 in]
                }
              }
            }
            n14 = New Data Value Reference(data value=w39) -> (data value reference=w51:refnum<data-value>)  [unwired: 1 in, 1 out]
            n15 = New Data Value Reference(data value=w38) -> (data value reference=w50:refnum<data-value>)  [unwired: 1 in, 1 out]
            n16 = New Data Value Reference(data value=w43) -> (data value reference=w49:refnum<data-value>)  [unwired: 1 in, 1 out]
            n17 = New Data Value Reference(data value=w42) -> (data value reference=w54:refnum<data-value>)  [unwired: 1 in, 1 out]
            n18 = New Data Value Reference(data value=w41) -> (data value reference=w53:refnum<data-value>)  [unwired: 1 in, 1 out]
            n19 = New Data Value Reference(data value=w40) -> (data value reference=w52:refnum<data-value>)  [unwired: 1 in, 1 out]
          }
          frame 1 {
            # "Set some plot settings (color tables, scan names, )"
            # "Skip or don't skip filtering step"
            # "Set color tables"
            n20 = Transpose 2D Array(2D array=w102) -> (transposed array=w105:dbl[][])
            n21 = local read "Scan names 2"() -> (w89:string[])
            n22 = for {
              tunnel: w105 -> [w115] mode=indexing
              tunnel: [w116] -> _ mode=indexing
              tunnel: w101 -> [w112]
              shift-right: [w113] -> w83
              shift-left: dbl[] [] -> [w114]
              shift-right: [w111] -> w82
              shift-left: dbl[] [] -> [w110]
              n23 = Build Array (concatenate)(w114, w115) -> (w113:dbl[])
              n24 = Build Array (concatenate)(w110, w112) -> (w111:dbl[])
              n25 = Bundle(w115, "Vslow"=w112) -> (w116:cluster{dbl[], "Vslow":dbl[]})  [unwired: 1 in]
            }
            n26 = Index Array(array=w89, index #2=1 ("index")) -> (element #1=w87:string, element #2=w86:string)  [unwired: 1 in]
            n27 = property on="XY Graph" class="XYGraph (strict)"("XScale.NameLbl.Text"=w87) -> ()  [unwired: 2 in, 2 out]
            n28 = property on="XY Graph" class="XYGraph (strict)"("YScale.NameLbl.Text"=w86) -> ()  [unwired: 2 in, 2 out]
            n29 = Bundle(w83, w82) -> (w81:cluster{dbl[], dbl[]})  [unwired: 1 in]
            "XY Graph" <- w81
            n30 = disable-structure shown="Disabled" {
              disable-tunnel: w81 -> [w106 _]
              frame Disabled {
                n31 = for {
                  tunnel: w106 -> [_]
                  i -> [w107]
                  n32 = stacked-sequence {
                    tunnel: w107 -> [w108 _]
                    frame #0 {
                      n33 = property on="XY Graph" class="XYGraph (strict)"("Active Plot"=w108) -> ()  [unwired: 2 in, 2 out]
                    }
                    frame #1 {
                      n34 = property on="XY Graph" class="XYGraph (strict)"("Plot.Point Style"=u8 13) -> ()  [unwired: 2 in, 2 out]
                    }
                  }
                }
              }
              frame Enabled {
              }
            }
            n35 = Select(t=2, s="Filter retrieved data?", f=3) -> (s? t:f=w91:i32)
            n36 = Reverse 1D Array(array="color scale") -> (reversed array=w96:u32[])
            n37 = call <userlib>:"Make Color Table.vi"("Array"=w96) -> ("Color Tbl"=w95:u32[])  [unwired: 1 in, 3 out]
            n38 = property on="Intensity Graph" class="IntGraph (strict)"("Color Table"=w95) -> ()  [unwired: 2 in, 2 out]
            n39 = property on="2 term trans" class="IntGraph (strict)"("Color Table"=w95) -> ()  [unwired: 2 in, 2 out]
            n40 = property on="Intensity Graph 2" class="IntGraph (strict)"("Color Table"=w95) -> ()  [unwired: 2 in, 2 out]
            n41 = property on="2term Intensity" class="IntGraph (strict)"("Color Table"=w95) -> ()  [unwired: 2 in, 2 out]
          }
          frame 2 {
            # "Filter data (Savitsky-Golay)"
            n42 = in-place {
              n43 = in-place-dvr #1(w124) -> (w170:T8)  [unwired: 1 out]
              n44 = in-place-dvr #2(w123) -> (w169:T8)  [unwired: 1 out]
              n45 = stacked-sequence {
                tunnel: w170 -> [w174 _]
                tunnel: [w173 _] -> w168
                tunnel: [_ w189] -> w167
                tunnel: "side points 2T" -> [w172 w188]
                tunnel: w169 -> [_ w187]
                frame #0 {
                  n46 = for {
                    tunnel: [w177] -> w173 mode=indexing
                    tunnel: w174 -> [w176] mode=indexing
                    tunnel: w172 -> [w175]
                    n47 = for {
                      tunnel: [w180] -> w177 mode=indexing
                      tunnel: w176 -> [w179] mode=indexing
                      tunnel: w175 -> [w178]
                      n48 = for {
                        tunnel: [w183] -> w180 mode=indexing
                        tunnel: w179 -> [w182] mode=indexing
                        tunnel: w178 -> [w181]
                        n49 = Unbundle(w182) -> ("Decimated Array"=w184:dbl[], "Decimated Array"=w186:dbl[])
                        n50 = call-poly <vilib>:"Savitzky-Golay Filter.vi"("side points"=w181, "X"=w186) -> ("Filtered X"=w185:dbl[])  [unwired: 8 in, 1 out]
                        n51 = Bundle("Decimated Array"=w184, "Filtered X"=w185) -> (w183:T9)  [unwired: 1 in]
                        "side points 2Ttemp" <- w181
                      }
                    }
                  }
                }
                frame #1 {
                  n52 = for {
                    tunnel: [w192] -> w189 mode=indexing
                    tunnel: w188 -> [w191]
                    tunnel: w187 -> [w190] mode=indexing
                    n53 = for {
                      tunnel: [w195] -> w192 mode=indexing
                      tunnel: w191 -> [w194]
                      tunnel: w190 -> [w193] mode=indexing
                      n54 = for {
                        tunnel: [w196] -> w195 mode=indexing
                        tunnel: w194 -> [w201]
                        tunnel: w193 -> [w200] mode=indexing
                        n55 = Unbundle(w200) -> ("Decimated Array"=w197:dbl[], "Decimated Array"=w199:dbl[])
                        n56 = call-poly <vilib>:"Savitzky-Golay Filter.vi"("side points"=w201, "X"=w199) -> ("Filtered X"=w198:dbl[])  [unwired: 8 in, 1 out]
                        n57 = Bundle("Decimated Array"=w197, "Filtered X"=w198) -> (w196:T9)  [unwired: 1 in]
                      }
                    }
                  }
                }
              }
              n58 = in-place-dvr #1(w168) -> (w117:refnum<data-value>)  [unwired: 1 out]
              n59 = in-place-dvr #2(w167) -> (w122:refnum<data-value>)  [unwired: 1 out]
            }
            n60 = in-place {
              n61 = in-place-dvr #3(w121) -> (w135:T8)  [unwired: 1 out]
              n62 = in-place-dvr #4(w120) -> (w134:T8)  [unwired: 1 out]
              n63 = stacked-sequence {
                tunnel: w135 -> [w139 _]
                tunnel: [w138 _] -> w133
                tunnel: w134 -> [_ w154]
                tunnel: [_ w153] -> w132
                tunnel: "side points 4T" -> [_ w152]
                tunnel: "side points 4T" -> [w137 _]
                frame #0 {
                  n64 = for {
                    tunnel: [w142] -> w138 mode=indexing
                    tunnel: w139 -> [w141] mode=indexing
                    tunnel: w137 -> [w140]
                    n65 = for {
                      tunnel: [w145] -> w142 mode=indexing
                      tunnel: w141 -> [w144] mode=indexing
                      tunnel: w140 -> [w143]
                      n66 = for {
                        tunnel: [w148] -> w145 mode=indexing
                        tunnel: w144 -> [w147] mode=indexing
                        tunnel: w143 -> [w146]
                        n67 = Unbundle(w147) -> ("Decimated Array"=w149:dbl[], "Decimated Array"=w151:dbl[])
                        n68 = call-poly <vilib>:"Savitzky-Golay Filter.vi"("side points"=w146, "X"=w151) -> ("Filtered X"=w150:dbl[])  [unwired: 8 in, 1 out]
                        n69 = Bundle("Decimated Array"=w149, "Filtered X"=w150) -> (w148:T9)  [unwired: 1 in]
                      }
                    }
                  }
                }
                frame #1 {
                  n70 = for {
                    tunnel: [w157] -> w153 mode=indexing
                    tunnel: w154 -> [w156] mode=indexing
                    tunnel: w152 -> [w155]
                    n71 = for {
                      tunnel: [w160] -> w157 mode=indexing
                      tunnel: w156 -> [w159] mode=indexing
                      tunnel: w155 -> [w158]
                      n72 = for {
                        tunnel: [w163] -> w160 mode=indexing
                        tunnel: w159 -> [w162] mode=indexing
                        tunnel: w158 -> [w161]
                        n73 = Unbundle(w162) -> ("Decimated Array"=w164:dbl[], "Decimated Array"=w166:dbl[])
                        n74 = call-poly <vilib>:"Savitzky-Golay Filter.vi"("side points"=w161, "X"=w166) -> ("Filtered X"=w165:dbl[])  [unwired: 8 in, 1 out]
                        n75 = Bundle("Decimated Array"=w164, "Filtered X"=w165) -> (w163:T9)  [unwired: 1 in]
                        "side points 4Ttemp" <- w161
                      }
                    }
                  }
                }
              }
              n76 = in-place-dvr #3(w133) -> (w119:refnum<data-value>)  [unwired: 1 out]
              n77 = in-place-dvr #4(w132) -> (w118:refnum<data-value>)  [unwired: 1 out]
            }
          }
          frame 3 {
            n78 = in-place {
              in-place-border: w218 -> [w250]
              in-place-border: w217 -> [w248]
              in-place-border: [w232] -> w216
              in-place-border: [FALSE] -> w215
              in-place-border: w214 -> [w227]
              w246 = dbl[] []
              # "Vslow VALUES"
              # "find INDEX of crosshairs Y value in Vslow arr"
              # "runs \"#Vslow\" # of times bc thats # of rows in Vfast (each row = Vfast values)"
              # "slow INDICES"
              # "Cursor X location (INDEX) (array for some reason)"
              # "fast"
              # "slow"
              # "ex. BG value"
              # "#TODO: find out what this does\nfinds fast index of cursor X position"
              n79 = in-place-dvr #5(w208) -> (w219:T8)  [unwired: 1 out]
              n80 = in-place-dvr #6(w207) -> (w220:T8)  [unwired: 1 out]
              n81 = in-place-dvr #7(w213) -> (w221:T8)  [unwired: 1 out]
              n82 = in-place-dvr #8(w211) -> (w222:T8)  [unwired: 1 out]
              n83 = in-place-dvr #9(w210) -> (w224:T8)  [unwired: 1 out]
              n84 = in-place-dvr #10(w209) -> (w223:T8)  [unwired: 1 out]
              n85 = local read "Field/Temperature"() -> (w229:i32)
              n86 = property on="XY Graph" class="XYGraph (strict)" props=["Cursor", "Cursor Position", "Cursor", "Cursor X", "Cursor", "Cursor Y"]() -> ("Cursor.Cursor X"=w247:dbl, "Cursor.Cursor Y"=w252:dbl)  [unwired: 2 in, 3 out]
              "Field" <- w252
              n87 = Array Size(array=w227) -> (size(s)=w226:i32)
              n88 = Decrement(x=w226) -> (x-1=w225:i32)
              n89 = property on="Field/Temperature" class="Slide (strict)"("Scale.Maximum"=w225) -> ()  [unwired: 2 in, 2 out]
              n90 = Index Array(array=w227, index=w229) -> (element=→"slowest":dbl)
              n91 = call <vilib>:"Search Ordered Table.vi"("x value"=w252, "ordered x array"=w250) -> ("fractional index"=w251:dbl)  [unwired: 9 in]
              n92 = Round To Nearest(number=w251) -> (nearest integer value=w249:dbl)
              n93 = for {
                tunnel: w248 -> [w272] mode=indexing
                tunnel: w247 -> [w271]
                shift-right: [w262] -> w244
                shift-left: w246 -> [w261]
                shift-right: [w257] -> w245
                shift-left: w246 -> [w256]
                i -> [w260]
                n94 = Subtract(x=w271, y=w272) -> (x-y=w276:dbl[])
                n95 = Index Array(array=w272, index #1=0 ("index"), index #2=1 ("index")) -> (element #1=w269:dbl, element #2=w268:dbl)
                n96 = Absolute Value(x=w276) -> (abs(x)=w275:dbl[])
                n97 = Subtract(x=w269, y=w268) -> (x-y=w274:dbl)
                n98 = Absolute Value(x=w274) -> (abs(x)=w267:dbl)
                n99 = Array Max & Min(array=w275) -> (min value=w264:dbl, min index (indices)=w255:i32)  [unwired: 2 out]
                n100 = Divide(x=w267, y=2.0) -> (x/y=w265:dbl)
                n101 = Less?(x=w265, y=w264) -> (x < y?=w258:bool)
                n102 = Build Array (concatenate)(w261, w255) -> (w263:dbl[])
                n103 = Build Array (concatenate)(w256, w260) -> (w259:dbl[])
                n104 = Select(t=w256, s=w258, f=w259) -> (s? t:f=w257:dbl[])
                n105 = Select(t=w261, s=w258, f=w263) -> (s? t:f=w262:dbl[])
              }
              n106 = local read "side points 4Ttemp"() -> (w241:i32)
              n107 = local read "side points 2Ttemp"() -> (w242:i32)
              n108 = local read "side points 2T"() -> (w243:i32)
              n109 = local read "side points 4T"() -> (w240:i32)
              n110 = Not Equal?(x=w241, y=w240) -> (x != y?=w239:bool)
              n111 = Not Equal?(x=w243, y=w242) -> (x != y?=w238:bool)
              n112 = Or(x=w239, y=w238) -> (x .or. y?=w237:bool)
              n113 = Select(t=2, s=w237, f=3) -> (s? t:f=w230:i32)
              n114 = Select(t=4, s="stop", f=w230) -> (s? t:f=w232:i32)
              n115 = case shown="\"2 terminal R vs I\"" "Tab Control" {
                tunnel: w220 -> [_ _ w294 w317 w338 _ _ _ _ _ _]
                tunnel: "Field/Temperature" -> [_ _ w285 w322 _ w436 w504 w614 w694 _ _]
                tunnel: w249 -> [_ _ w284 _ w346 w438 w492 w618 w698 w741 _]
                tunnel: w224 -> [_ _ w292 w320 w340 w437 _ _ _ _ _]
                tunnel: w219 -> [_ _ w289 w313 w339 _ _ _ _ _ _]
                tunnel: w221 -> [_ _ w286 w323 w344 _ w528 _ _ w717 _]
                tunnel: w222 -> [_ _ w283 _ _ _ w505 _ w674 _ w843]
                tunnel: w223 -> [_ _ w287 _ _ _ _ w596 _ _ _]
                tunnel: w248 -> [_ _ _ _ w347 w427 w540 w608 w689 w743 _]
                tunnel: w250 -> [_ _ _ _ _ _ _ w570 _ w735 _]
                tunnel: w227 -> [_ _ _ _ _ _ _ _ _ _ _]
                tunnel: w247 -> [_ _ _ _ _ _ _ _ _ _ _]
                tunnel: w245 -> [_ _ _ w315 _ w435 w544 w613 w693 _ _]
                tunnel: w244 -> [_ _ _ w314 _ w434 w543 w612 w692 _ _]
                frame "Device ", Default {
                }
                frame "Data generation" {
                }
                frame "Vary Vfast" {
                  # "shows plots for all values of Vfast, while the cursor varies Vslow"
                  n116 = Index Array(array=w289, index (dim 0)=w285) -> (element=w290:T10)  [unwired: 2 in]
                  n117 = Index Array(array=w294, index (dim 0)=w285) -> (element=w293:T10)  [unwired: 2 in]
                  n118 = Index Array(array=w286, index (dim 0)=w285) -> (element=w288:T10)  [unwired: 2 in]
                  n119 = Index Array(array=w283, index (dim 0)=w285, index (dim 1)=w284) -> (element=w279:T11)  [unwired: 1 in]
                  "dV/dI 2T" <- w279
                  n120 = Index Array(array=w292, index (dim 0)=w285) -> (element=w291:T10)  [unwired: 2 in]
                  n121 = Index Array(array=w287, index (dim 0)=w285, index (dim 1)=w284) -> (element=w281:T11)  [unwired: 1 in]
                  "dV/dI vs I" <- w281
                  n122 = Index Array(array=w291, index (row)=w284) -> (element=w280:T11)  [unwired: 1 in]
                  "dI/dV vs V" <- w280
                  n123 = Index Array(array=w290, index (row)=w284) -> (element=w282:T11)  [unwired: 1 in]
                  "IV 2T" <- w282
                  n124 = Index Array(array=w293, index (row)=w284) -> (element=w277:T11)  [unwired: 1 in]
                  "IV" <- w277
                  n125 = Index Array(array=w288, index (row)=w284) -> (element=w278:T11)  [unwired: 1 in]
                  "dI/dV 2T" <- w278
                  n126 = for {
                    tunnel: w282 -> [w312] mode=indexing
                    tunnel: [w311] -> _ mode=indexing
                    tunnel: [w310] -> _ mode=indexing
                    n127 = Unbundle(w312) -> ("Decimated Array"=w311:dbl[], "Decimated Array"=w310:dbl[])
                  }
                  n128 = for {
                    tunnel: w277 -> [w309] mode=indexing
                    tunnel: [w308] -> _ mode=indexing
                    tunnel: [w307] -> _ mode=indexing
                    n129 = Unbundle(w309) -> ("Decimated Array"=w308:dbl[], "Decimated Array"=w307:dbl[])
                  }
                  n130 = for {
                    tunnel: w278 -> [w306] mode=indexing
                    tunnel: [w305] -> _ mode=indexing
                    tunnel: [w304] -> _ mode=indexing
                    n131 = Unbundle(w306) -> ("Decimated Array"=w305:dbl[], "Decimated Array"=w304:dbl[])
                  }
                  n132 = for {
                    tunnel: w279 -> [w303] mode=indexing
                    tunnel: [w302] -> _ mode=indexing
                    tunnel: [w301] -> _ mode=indexing
                    n133 = Unbundle(w303) -> ("Decimated Array"=w302:dbl[], "Decimated Array"=w301:dbl[])
                  }
                  n134 = for {
                    tunnel: w280 -> [w300] mode=indexing
                    tunnel: [w299] -> _ mode=indexing
                    tunnel: [w298] -> _ mode=indexing
                    n135 = Unbundle(w300) -> ("Decimated Array"=w299:dbl[], "Decimated Array"=w298:dbl[])
                  }
                  n136 = for {
                    tunnel: w281 -> [w297] mode=indexing
                    tunnel: [w296] -> _ mode=indexing
                    tunnel: [w295] -> _ mode=indexing
                    n137 = Unbundle(w297) -> ("Decimated Array"=w296:dbl[], "Decimated Array"=w295:dbl[])
                  }
                }
                frame "Vary Vslow" {
                  # "shows plots for all values of Vslow, while the cursor varies Vfast"
                  n138 = for {
                    tunnel: w323 -> [w334]
                    tunnel: w322 -> [w327]
                    tunnel: w314 -> [w325] mode=indexing
                    tunnel: [w333] -> w321 mode=indexing
                    tunnel: w315 -> [w326] mode=indexing
                    tunnel: w320 -> [w332]
                    tunnel: [w331] -> w319 mode=indexing
                    tunnel: w313 -> [w330]
                    tunnel: [w329] -> w318 mode=indexing
                    tunnel: w317 -> [w328]
                    tunnel: [w324] -> w316 mode=indexing
                    n139 = Index Array(array=w328, index (dim 0)=w327, index (dim 1)=w326, index (dim 2)=w325) -> (element=w324:T7)
                    n140 = Index Array(array=w330, index (dim 0)=w327, index (dim 1)=w326, index (dim 2)=w325) -> (element=w329:T7)
                    n141 = Index Array(array=w332, index (dim 0)=w327, index (dim 1)=w326, index (dim 2)=w325) -> (element=w331:T7)
                    n142 = Index Array(array=w334, index (dim 0)=w327, index (dim 1)=w326, index (dim 2)=w325) -> (element=w333:T7)
                  }
                  "IV slow 4T" <- w316
                  "dI/dV slow 4T" <- w319
                  "dI/dV slow 2T" <- w321
                  "IV slow 2T" <- w318
                }
                frame "Vary Fields" {
                  n143 = for {
                    tunnel: w347 -> [w359] mode=indexing
                    tunnel: w346 -> [w358]
                    tunnel: [w359] -> w345
                    i -> [w361]
                    n144 = To Long Integer(number=w358) -> (32bit integer=w365:i32)
                    n145 = Subtract(x=w359, y=w359) -> (x-y=w364:dbl[])
                    n146 = Absolute Value(x=w364) -> (abs(x)=w363:dbl[])
                    n147 = Equal?(x=w365, y=w361) -> (x = y?=w360:bool)
                    n148 = Array Max & Min(array=w363) -> (min index (indices)=w362:i32)  [unwired: 3 out]
                    n149 = case shown="True" w360 {
                      tunnel: w362 -> [_ w367]
                      tunnel: w358 -> [_ w366]
                      frame False {
                      }
                      frame True {
                        "Vslow index" <- w367
                        "Vfast index" <- w366
                      }
                    }
                  }
                  n150 = local read "Vfast index"() -> (w343:dbl)
                  n151 = local read "Vslow index"() -> (w342:i32)
                  n152 = flat-sequence {
                    tunnel: w345 -> [_]
                    tunnel: w344 -> [w357]
                    tunnel: w343 -> [w351]
                    tunnel: w342 -> [w352]
                    tunnel: [w356] -> w341
                    tunnel: w340 -> [w355]
                    tunnel: w339 -> [w354]
                    tunnel: w338 -> [w353]
                    tunnel: [w350] -> w337
                    tunnel: [w349] -> w336
                    tunnel: [w348] -> w335
                    frame #0 {
                      n153 = Index Array(array=w353, index (dim 1)=w351, index (dim 2)=w352) -> (element=w349:T11)  [unwired: 1 in]
                      n154 = Index Array(array=w357, index (dim 1)=w351, index (dim 2)=w352) -> (element=w356:T11)  [unwired: 1 in]
                      n155 = Index Array(array=w355, index (dim 1)=w351, index (dim 2)=w352) -> (element=w348:T11)  [unwired: 1 in]
                      n156 = Index Array(array=w354, index (dim 1)=w351, index (dim 2)=w352) -> (element=w350:T11)  [unwired: 1 in]
                    }
                  }
                  "dI/dV vary 3rd 4T" <- w335
                  "dI/dV vary 3rd 2T" <- w341
                  "IV vary 3rd 4T" <- w336
                  "IV vary 3rd 2T" <- w337
                }
                frame "4 terminal G vs V" {
                  w413 = 3.874e-05
                  # "idk wot plot this is"
                  n157 = Index Array(array=w427, index (row)=w438) -> (element=w394:dbl[])  [unwired: 1 in]
                  n158 = Index Array(array=w437, index (dim 0)=w436, index (dim 1)=w438) -> (element=w410:T11)  [unwired: 1 in]
                  n159 = for {
                    tunnel: w437 -> [w476]
                    tunnel: w436 -> [w475]
                    tunnel: w435 -> [w470] mode=indexing
                    tunnel: w434 -> [w471] mode=indexing
                    tunnel: [w474] -> w433 mode=indexing
                    tunnel: w427 -> [w473]
                    tunnel: [w472] -> w421 mode=indexing
                    tunnel: "X Step" -> [w468]
                    tunnel: "X High" -> [w467]
                    tunnel: "X Low" -> [w466]
                    n160 = Index Array(array=w473, index (row)=w471, index (col)=w470) -> (element=w472:dbl)
                    n161 = Index Array(array=w476, index (dim 0)=w475, index (dim 1)=w470, index (dim 2)=w471) -> (element=w469:T7)
                    n162 = call <userlib>:"Decimate_VS_X_Value.vi"("XY Graph kind 1"=w469, "X Step"=w468, "X High"=w467, "X Low"=w466) -> ("Interpolated"=w465:cluster{dbl[], dbl[]})  [unwired: 6 in, 1 out]
                    n163 = Unbundle(w465) -> (w474:dbl[])  [unwired: 1 out]
                  }
                  n164 = for {
                    tunnel: [w482] -> _ mode=indexing
                    tunnel: [w484] -> w441
                    tunnel: [w479] -> w442
                    tunnel: [w485] -> w384
                    tunnel: w410 -> [w483] mode=indexing
                    tunnel: [w482] -> w409 mode=indexing
                    tunnel: "X Low" -> [w481]
                    tunnel: "X High" -> [w480]
                    tunnel: "X Step" -> [w479]
                    tunnel: "Voffset-4T" -> [w478]
                    n165 = Subtract(x=w481, y=w478) -> (x-y=w484:dbl)
                    n166 = call <userlib>:"Decimate_VS_X_Value.vi"("fake point value"="fake point value", "XY Graph kind 1"=w483, "X Step"=w479, "X High"=w480, "X Low"=w481) -> ("Interpolated"=w487:cluster{dbl[], dbl[]})  [unwired: 5 in, 1 out]
                    n167 = Unbundle(w487) -> (w486:dbl[], w482:dbl[])
                    n168 = Subtract(x=w486, y=w478) -> (x-y=w485:dbl[])
                  }
                  n169 = Index Array(array=w394, index #1=0 ("index"), index #2=1 ("index")) -> (element #1=w397:dbl, element #2=w395:dbl)
                  n170 = Subtract(x=w395, y=w397) -> (x-y=w398:dbl)
                  n171 = case shown="True" "No scale?" {
                    tunnel: "Breakdown High" -> [_ w447]
                    tunnel: "Breakdown Low" -> [_ w448]
                    tunnel: w398 -> [w445 _]
                    tunnel: w397 -> [w444 w454]
                    tunnel: [w445 w450] -> w370
                    tunnel: [w444 w451] -> w371
                    tunnel: w395 -> [_ w453]
                    tunnel: w394 -> [w443 w449]
                    tunnel: [w443 w446] -> w369
                    frame False {
                    }
                    frame True {
                      n172 = call <userlib>:"Scale Voltage.vi"("Scale factor"=w453, "Breakdown Low"=w448, "Breakdown High"=w447) -> ("Real Voltage"=w452:dbl)
                      n173 = call <userlib>:"Scale Voltage.vi"("Scale factor"=w454, "Breakdown Low"=w448, "Breakdown High"=w447) -> ("Real Voltage"=w451:dbl)
                      n174 = Subtract(x=w452, y=w451) -> (x-y=w450:dbl)
                      n175 = for {
                        tunnel: w449 -> [w458] mode=indexing
                        tunnel: w448 -> [w457]
                        tunnel: w447 -> [w456]
                        tunnel: [w455] -> w446 mode=indexing
                        n176 = call <userlib>:"Scale Voltage.vi"("Scale factor"=w458, "Breakdown Low"=w457, "Breakdown High"=w456) -> ("Real Voltage"=w455:dbl)
                      }
                    }
                  }
                  n177 = Transpose 2D Array(2D array=w433) -> (transposed array=w432:dbl[][])
                  n178 = Transpose 2D Array(2D array=w409) -> (transposed array=w429:dbl[][])
                  n179 = case shown="True" "Log scale?" {
                    tunnel: w432 -> [w462 w464]
                    tunnel: [w462 w463] -> w431
                    frame False {
                    }
                    frame True {
                      n180 = Logarithm Base 10(1:w464) -> (0:w463:dbl[][])
                    }
                  }
                  "Intensity Graph 2" <- w431
                  n181 = Index Array(array=w421, index #1=0 ("index"), index #2=1 ("index")) -> (element #1=w425:dbl, element #2=w424:dbl)
                  n182 = case shown="True" "Log scale?" {
                    tunnel: w429 -> [w459 w461]
                    tunnel: [w459 w460] -> w378
                    frame False {
                    }
                    frame True {
                      n183 = Logarithm Base 10(1:w461) -> (0:w460:dbl[][])
                    }
                  }
                  "Intensity Graph" <- w378
                  n184 = Subtract(x=w424, y=w425) -> (x-y=w426:dbl)
                  n185 = Bundle(w425, w426) -> (w420:cluster{dbl, dbl})  [unwired: 1 in]
                  n186 = call "transcond_intensity_v2.vi"("derivative bin size"="derivative bin size", "Conductance"=w378) -> ("Transconductance"=w380:dbl[][])  [unwired: 9 in]
                  "Transconductance" <- w380
                  n187 = property on="Intensity Graph 2" class="IntGraph (strict)"("YScale.Ofst&Mult"=w420) -> ()  [unwired: 2 in, 2 out]
                  n188 = Index Array(array=w378) -> (element=w377:dbl[])  [unwired: 2 in]
                  n189 = property on="Intensity Graph" class="IntGraph (strict)"() -> ("Cursor.Cursor Plot"=w415:i32)  [unwired: 2 in, 2 out]
                  n190 = Index Array(array=w380) -> (element=w379:dbl[])  [unwired: 2 in]
                  n191 = Bundle("Real Voltage"=w371, w370) -> (w381:cluster{"Real Voltage":dbl, dbl})  [unwired: 1 in]
                  "Y scale" <- w381
                  n192 = Array Size(array=w377) -> (size(s)=w375:i32)
                  n193 = local read "Scan names 2"() -> (w408:string[])
                  n194 = property on="Intensity Graph" class="IntGraph (strict)"("YScale.Ofst&Mult"=w381) -> ()  [unwired: 2 in, 2 out]
                  n195 = Array Size(array=w379) -> (size(s)=w376:i32)
                  n196 = Index Array(array=w378, index (col)=w415) -> (element=w414:dbl[])  [unwired: 1 in]
                  n197 = Divide(x=w375, y=w376) -> (x/y=w374:dbl)
                  n198 = Multiply(x=w370, y=w374) -> (x*y=w373:dbl)
                  n199 = Index Array(array=w408, index #2=1 ("index")) -> (element #1=w405:string, element #2=w406:string)  [unwired: 1 in]
                  n200 = Divide(x=w414, y=w413) -> (x/y=w418:dbl[])
                  n201 = property on="Transconductance" class="IntGraph (strict)"() -> ("Cursor.Cursor Index"=w383:i32)  [unwired: 2 in, 2 out]
                  n202 = property on="Transconductance" class="IntGraph (strict)"() -> ("Cursor.Cursor Plot"=w391:i32)  [unwired: 2 in, 2 out]
                  n203 = property on="Intensity Graph 2" class="IntGraph (strict)"("YScale.NameLbl.Text"=w406) -> ()  [unwired: 2 in, 2 out]
                  n204 = property on="Intensity Graph" class="IntGraph (strict)"("YScale.NameLbl.Text"=w405) -> ()  [unwired: 2 in, 2 out]
                  n205 = Bundle("Real Voltage"=w371, w373) -> (w372:cluster{"Real Voltage":dbl, dbl})  [unwired: 1 in]
                  n206 = Bundle(w384, w418) -> (→"X line cut 2":cluster{dbl[], dbl[]})  [unwired: 1 in]
                  n207 = property on="Intensity Graph" class="IntGraph (strict)"() -> ("Cursor.Cursor Index"=w417:i32)  [unwired: 2 in, 2 out]
                  n208 = Index Array(array=w380, index (col) #1=w391, index (row) #2=w383) -> (element #1=w390:dbl[], element #2=w382:dbl[])  [unwired: 2 in]
                  n209 = Bundle(w384, "Transconductance"=w390) -> (w389:cluster{dbl[], "Transconductance":dbl[]})  [unwired: 1 in]
                  "X line cut 3" <- w389
                  n210 = Bundle(w441, "X Step"=w442) -> (w392:cluster{dbl, "X Step":dbl})  [unwired: 1 in]
                  "X scale" <- w392
                  n211 = Index Array(array=w378, index (row)=w417) -> (element=w416:dbl[])  [unwired: 1 in]
                  n212 = Divide(x=w416, y=w413) -> (x/y=w419:dbl[])
                  n213 = property on="Transconductance" class="IntGraph (strict)"() -> ("XScale.Maximum"=w386:dbl, "XScale.Minimum"=w387:dbl)  [unwired: 2 in, 2 out]
                  n214 = Bundle("Vfast"=w369, "Transconductance"=w382) -> (→"Y line cut 8":cluster{"Vfast":dbl[], "Transconductance":dbl[]})  [unwired: 1 in]
                  n215 = Bundle("Vfast"=w369, w419) -> (→"Y line cut 2":cluster{"Vfast":dbl[], dbl[]})  [unwired: 1 in]
                  n216 = property on="Intensity Graph 2" class="IntGraph (strict)"("XScale.Ofst&Mult"=w392) -> ()  [unwired: 2 in, 2 out]
                  n217 = property on="Intensity Graph" class="IntGraph (strict)"("XScale.Ofst&Mult"=w392) -> ()  [unwired: 2 in, 2 out]
                  n218 = property on="Transconductance" class="IntGraph (strict)"("XScale.Ofst&Mult"=w392, "YScale.Ofst&Mult"=w372) -> ()  [unwired: 2 in, 2 out]
                  n219 = Build Array(w389) -> (w388:cluster{dbl[], "Transconductance":dbl[]}[])
                  n220 = call "Restrict X Domain of Graph_retrieve program.vi"("XY Graph"=w388, "X Scale.Range:Maximum"=w386, "X Scale.Range:Minimum"=w387) -> ("Cluster"=→"X line cut 7":cluster{dbl[], dbl[]})  [unwired: 1 out]
                }
                frame "2 terminal G vs V" {
                  w490 = T12 {"X Low 2T"=0.0, "X High 2T"=0.0, "X Step 2T"=0.0, "Voffset -2T"=0.0}  # Decimate Controls
                  # "outputs Vfast values"
                  # "B ind"
                  # "all the same xpos ind"
                  # "0-7"
                  # "#TODO: Figure out what this for loop does.."
                  n221 = Index Array(array=w505, index (dim 0)=w504, index (dim 1)=w492) -> (element=w503:T11)  [unwired: 1 in]
                  n222 = Index Array(array=w528, index (dim 0)=w504, index (dim 1)=w492) -> (element=w521:T11)  [unwired: 1 in]
                  n223 = for {
                    tunnel: w528 -> [w569]
                    tunnel: w504 -> [w568]
                    tunnel: w544 -> [w564] mode=indexing
                    tunnel: w543 -> [w563] mode=indexing
                    tunnel: [w567] -> w542 mode=indexing
                    tunnel: w540 -> [w566]
                    tunnel: [w565] -> w534 mode=indexing
                    tunnel: "X Step 2T" -> [w560]
                    tunnel: "X High 2T" -> [w559]
                    tunnel: "X Low 2T" -> [w558]
                    n224 = Index Array(array=w566, index (row)=w563, index (col)=w564) -> (element=w565:dbl)
                    n225 = Index Array(array=w569, index (dim 0)=w568, index (dim 1)=w564, index (dim 2)=w563) -> (element=w562:T7)
                    n226 = call <userlib>:"Decimate_VS_X_Value.vi"("XY Graph kind 1"=w562, "X Step"=w560, "X High"=w559, "X Low"=w558) -> ("Interpolated"=w561:cluster{dbl[], dbl[]})  [unwired: 6 in, 1 out]
                    n227 = Unbundle(w561) -> (w567:dbl[])  [unwired: 1 out]
                  }
                  n228 = for {
                    tunnel: w503 -> [w552] mode=indexing
                    tunnel: [w551] -> w500 mode=indexing
                    tunnel: [w550] -> _ mode=indexing
                    # "current"
                    n229 = Unbundle(w552) -> ("Decimated Array"=w551:dbl[], "Decimated Array"=w550:dbl[])
                  }
                  n230 = local read "Scan names 2"() -> (w520:string[])
                  n231 = Bundle(cluster=w490, "X Low 2T"="X Low 2T", "X High 2T"="X High 2T", "X Step 2T"="X Step 2T", "Voffset -2T"="Voffset -2T") -> (w495:T12)
                  n232 = Index Array(array=w520, index #2=1 ("index")) -> (element #1=w517:string, element #2=w518:string)  [unwired: 1 in]
                  n233 = Transpose 2D Array(2D array=w500) -> (transposed array=→"2term Intensity Current vs. Voltage":dbl[][])
                  n234 = call "DataVIS_Decimate+Fill_Intensity_Plot.vi"("Log Scale (T)"="Log scale?", "fake point value"="fake point value 2", "Decimate Controls"=w495, "X and Y Arrays to decimate"=w521) -> ("Offset X Low"=w494:dbl, "Decimated X values"=w510:dbl[], "Arr of Y arrays (intensity info)"=w488:dbl[][])  [unwired: 4 in, 1 out]
                  "2term Intensity" <- w488
                  n235 = property on="2 term trans" class="IntGraph (strict)"("YScale.NameLbl.Text"=w518) -> ()  [unwired: 2 in, 2 out]
                  n236 = property on="2term Intensity" class="IntGraph (strict)"("YScale.NameLbl.Text"=w517) -> ()  [unwired: 2 in, 2 out]
                  n237 = Index Array(array=w540, index (row)=w492) -> (element=w508:dbl[])  [unwired: 1 in]
                  n238 = Transpose 2D Array(2D array=w542) -> (transposed array=w541:dbl[][])
                  n239 = case shown="True" "Log scale?" {
                    tunnel: w541 -> [w555 w557]
                    tunnel: [w555 w556] -> _
                    frame False {
                    }
                    frame True {
                      n240 = Logarithm Base 10(1:w557) -> (0:w556:dbl[][])
                    }
                  }
                  n241 = Index Array(array=w508, index #1=0 ("index"), index #2=1 ("index")) -> (element #1=w546:dbl, element #2=w547:dbl)
                  n242 = Index Array(array=w534, index #1=0 ("index"), index #2=1 ("index")) -> (element #1=w538:dbl, element #2=w537:dbl)
                  n243 = case shown="True" "e^2/h?" {
                    tunnel: [1 3.874e-05] -> w529
                    frame False {
                    }
                    frame True {
                    }
                  }
                  n244 = Subtract(x=w537, y=w538) -> (x-y=w539:dbl)
                  n245 = Bundle("Offset X Low"=w494, "X Step 2T"="X Step 2T") -> (w502:cluster{"Offset X Low":dbl, "X Step 2T":dbl})  [unwired: 1 in]
                  n246 = Bundle(w538, w539) -> (w527:cluster{dbl, dbl})  [unwired: 1 in]
                  n247 = Subtract(x=w547, y=w546) -> (x-y=w545:dbl)
                  n248 = property on="2 term trans" class="IntGraph (strict)"("YScale.Ofst&Mult"=w527) -> ()  [unwired: 2 in, 2 out]
                  n249 = Bundle(w546, w545) -> (w501:cluster{dbl, dbl})  [unwired: 1 in]
                  n250 = property on="2term Intensity Current vs. Voltage" class="IntGraph (strict)"("XScale.Ofst&Mult"=w502, "YScale.Ofst&Mult"=w501) -> ()  [unwired: 2 in, 2 out]
                  n251 = property on="2term Intensity" class="IntGraph (strict)"("YScale.Ofst&Mult"=w501) -> ()  [unwired: 2 in, 2 out]
                  n252 = property on="2term Intensity" class="IntGraph (strict)"("XScale.Ofst&Mult"=w502) -> ()  [unwired: 2 in, 2 out]
                  n253 = property on="2 term trans" class="IntGraph (strict)"("XScale.Ofst&Mult"=w502) -> ()  [unwired: 2 in, 2 out]
                  n254 = property on="2term Intensity" class="IntGraph (strict)"() -> ("Cursor.Cursor Index"=w525:i32)  [unwired: 2 in, 2 out]
                  n255 = property on="2term Intensity" class="IntGraph (strict)"() -> ("Cursor.Cursor Plot"=w526:i32)  [unwired: 2 in, 2 out]
                  n256 = local read "derivative bin size"() -> (w516:dbl)
                  n257 = Index Array(array=w488, index (row)=w525) -> (element=w531:dbl[])  [unwired: 1 in]
                  n258 = Index Array(array=w488, index (col)=w526) -> (element=w530:dbl[])  [unwired: 1 in]
                  n259 = property on="2 term trans" class="IntGraph (strict)"() -> ("Cursor.Cursor Index"=w513:i32)  [unwired: 2 in, 2 out]
                  n260 = property on="2 term trans" class="IntGraph (strict)"() -> ("Cursor.Cursor Plot"=w514:i32)  [unwired: 2 in, 2 out]
                  n261 = call "transcond_intensity_v2.vi"("derivative bin size"=w516, "Conductance"=w488) -> ("Transconductance"=w515:dbl[][])  [unwired: 9 in]
                  "2 term trans" <- w515
                  n262 = Divide(x=w530, y=w529) -> (x/y=w532:dbl[])
                  n263 = Divide(x=w531, y=w529) -> (x/y=w533:dbl[])
                  n264 = Index Array(array=w515, index (col) #1=w514, index (row) #2=w513) -> (element #1=w512:dbl[], element #2=w511:dbl[])  [unwired: 2 in]
                  n265 = Bundle("Decimated X values"=w510, w532) -> (→"X line cut":cluster{"Decimated X values":dbl[], dbl[]})  [unwired: 1 in]
                  n266 = Bundle("Decimated X values"=w510, "Transconductance"=w512) -> (→"2term trans X line cut":T13)  [unwired: 1 in]
                  n267 = Bundle("Vfast"=w508, w533) -> (→"Y line cut":cluster{"Vfast":dbl[], dbl[]})  [unwired: 1 in]
                  n268 = Bundle("Vfast"=w508, "Transconductance"=w511) -> (→"2term trans Y line cut":cluster{"Vfast":dbl[], "Transconductance":dbl[]})  [unwired: 1 in]
                }
                frame "4 terminal R vs I" {
                  n269 = Index Array(array=w570, index #1=0 ("index"), index #2=1 ("index")) -> (element #1=w571:dbl, element #2=w606:dbl)
                  n270 = Subtract(x=w606, y=w571) -> (x-y=w607:dbl)
                  n271 = Bundle(w571, w607) -> (w599:cluster{dbl, dbl})  [unwired: 1 in]
                  n272 = Index Array(array=w608, index (row)=w618) -> (element=w573:dbl[])  [unwired: 1 in]
                  n273 = property on="Intensity Graph 6" class="IntGraph (strict)"("YScale.Ofst&Mult"=w599) -> ()  [unwired: 2 in, 2 out]
                  n274 = local read "Scan names 2"() -> (w592:string[])
                  n275 = Index Array(array=w573, index #1=0 ("index"), index #2=1 ("index")) -> (element #1=w616:dbl, element #2=w617:dbl)
                  n276 = Subtract(x=w617, y=w616) -> (x-y=w615:dbl)
                  n277 = Bundle(w616, w615) -> (w597:cluster{dbl, dbl})  [unwired: 1 in]
                  n278 = Index Array(array=w596, index (dim 0)=w614, index (dim 1)=w618) -> (element=w603:T11)  [unwired: 1 in]
                  n279 = Index Array(array=w592, index #2=1 ("index")) -> (element #1=w575:string, element #2=w574:string)  [unwired: 1 in]
                  n280 = property on="Y line cut 5" class="XYGraph (strict)"("XScale.NameLbl.Text"=w575) -> ()  [unwired: 2 in, 2 out]
                  n281 = property on="Y line cut 6" class="XYGraph (strict)"("XScale.NameLbl.Text"=w574) -> ()  [unwired: 2 in, 2 out]
                  n282 = property on="Intensity Graph 5" class="IntGraph (strict)"("YScale.NameLbl.Text"=w575) -> ()  [unwired: 2 in, 2 out]
                  n283 = for {
                    tunnel: [w643] -> w621
                    tunnel: [w645] -> w622
                    tunnel: [w642] -> w576
                    tunnel: w603 -> [w648] mode=indexing
                    tunnel: [w647] -> w602 mode=indexing
                    tunnel: "X Low 4t" -> [w643]
                    tunnel: "X High 4t" -> [w646]
                    tunnel: "X Step 4t" -> [w645]
                    tunnel: "fake point value 3" -> [w644]
                    n284 = call <userlib>:"Decimate_VS_X_Value.vi"("fake point value"=w644, "XY Graph kind 1"=w648, "X Step"=w645, "X High"=w646, "X Low"=w643) -> ("Interpolated"=w649:cluster{dbl[], dbl[]})  [unwired: 5 in, 1 out]
                    n285 = Unbundle(w649) -> (w642:dbl[], w647:dbl[])
                  }
                  n286 = property on="Intensity Graph 5" class="IntGraph (strict)"("YScale.Ofst&Mult"=w597) -> ()  [unwired: 2 in, 2 out]
                  n287 = for {
                    tunnel: w596 -> [w641]
                    tunnel: w614 -> [w640]
                    tunnel: w613 -> [w635] mode=indexing
                    tunnel: w612 -> [w636] mode=indexing
                    tunnel: [w639] -> w611 mode=indexing
                    tunnel: w608 -> [w638]
                    tunnel: [w637] -> _ mode=indexing
                    tunnel: "X Step 4t" -> [w634]
                    tunnel: "X High 4t" -> [w633]
                    tunnel: "X Low 4t" -> [w632]
                    tunnel: "fake point value 3" -> [w629]
                    n288 = Index Array(array=w638, index (row)=w636, index (col)=w635) -> (element=w637:dbl)
                    n289 = Index Array(array=w641, index (dim 0)=w640, index (dim 1)=w635, index (dim 2)=w636) -> (element=w631:T7)
                    n290 = call <userlib>:"Decimate_VS_X_Value.vi"("fake point value"=w629, "XY Graph kind 1"=w631, "X Step"=w634, "X High"=w633, "X Low"=w632) -> ("Interpolated"=w630:cluster{dbl[], dbl[]})  [unwired: 5 in, 1 out]
                    n291 = Unbundle(w630) -> (w639:dbl[])  [unwired: 1 out]
                  }
                  n292 = property on="Intensity Graph 6" class="IntGraph (strict)"("YScale.NameLbl.Text"=w574) -> ()  [unwired: 2 in, 2 out]
                  n293 = Transpose 2D Array(2D array=w602) -> (transposed array=w609:dbl[][])
                  n294 = Bundle("X Low 4t"=w621, "X Step 4t"=w622) -> (w598:cluster{"X Low 4t":dbl, "X Step 4t":dbl})  [unwired: 1 in]
                  n295 = Transpose 2D Array(2D array=w611) -> (transposed array=w610:dbl[][])
                  n296 = property on="Intensity Graph 6" class="IntGraph (strict)"("XScale.Ofst&Mult"=w598) -> ()  [unwired: 2 in, 2 out]
                  n297 = property on="Intensity Graph 5" class="IntGraph (strict)"("XScale.Ofst&Mult"=w598) -> ()  [unwired: 2 in, 2 out]
                  n298 = case shown="True" "Log scale? 2" {
                    tunnel: w610 -> [w626 w628]
                    tunnel: [w626 w627] -> w578
                    frame False {
                    }
                    frame True {
                      n299 = Logarithm Base 10(1:w628) -> (0:w627:dbl[][])
                    }
                  }
                  "Intensity Graph 6" <- w578
                  n300 = property on="Intensity Graph 5" class="IntGraph (strict)"() -> ("Cursor.Cursor Plot"=w586:i32, "Cursor.Cursor Index"=w587:i32)  [unwired: 2 in, 2 out]
                  n301 = case shown="True" "Log scale? 3" {
                    tunnel: w609 -> [w623 w625]
                    tunnel: [w623 w624] -> w588
                    frame False {
                    }
                    frame True {
                      n302 = Logarithm Base 10(1:w625) -> (0:w624:dbl[][])
                    }
                  }
                  "Intensity Graph 5" <- w588
                  n303 = call <userlib>:"GenerateLineCuts.vi"("X Array Y Cut"=w573, "Intensity Graph"=w588, "X Array X Cut"=w576, "width Y"="width Y 5", "Y Cursor (Cursor.Index)"=w587, "width X"="width X 5", "X Cursor (Cursor.Plot)"=w586) -> ("Y line cut"=→"Y line cut 5":cluster{"X Array Y Cut":dbl[], dbl[]}, "X line cut"=→"X line cut 5":cluster{"X Array X Cut":dbl[], dbl[]})  [unwired: 1 in, 2 out]
                  n304 = property on="Intensity Graph 6" class="IntGraph (strict)"() -> ("Cursor.Cursor Plot"=w585:i32, "Cursor.Cursor Index"=w577:i32)  [unwired: 2 in, 2 out]
                  n305 = call <userlib>:"GenerateLineCuts.vi"("X Array Y Cut"=w570, "Intensity Graph"=w578, "X Array X Cut"=w576, "width Y"="width Y 6", "Y Cursor (Cursor.Index)"=w577, "width X"="width X 6", "X Cursor (Cursor.Plot)"=w585) -> ("Y line cut"=→"Y line cut 6":cluster{"X Array Y Cut":dbl[], dbl[]}, "X line cut"=→"X line cut 6":cluster{"X Array X Cut":dbl[], dbl[]})  [unwired: 1 in, 2 out]
                }
                frame "2 terminal R vs I" {
                  w669 = 3.874e-05
                  n306 = Index Array(array=w689, index (row)=w698) -> (element=w665:dbl[])  [unwired: 1 in]
                  n307 = Index Array(array=w674, index (dim 0)=w694, index (dim 1)=w698) -> (element=w660:T11)  [unwired: 1 in]
                  n308 = Index Array(array=w665, index #1=0 ("index"), index #2=1 ("index")) -> (element #1=w696:dbl, element #2=w697:dbl)
                  n309 = Subtract(x=w697, y=w696) -> (x-y=w695:dbl)
                  n310 = local read "Scan names 2"() -> (w678:string[])
                  n311 = Bundle(w696, w695) -> (w682:cluster{dbl, dbl})  [unwired: 1 in]
                  n312 = property on="Intensity Graph 7" class="IntGraph (strict)"("YScale.Ofst&Mult"=w682) -> ()  [unwired: 2 in, 2 out]
                  n313 = Bundle("X Low 2t"="X Low 2t", "X High 2t"="X High 2t", "X Step 2t"="X Step 2t", "Voffset - 2T"="Voffset - 2T") -> (w659:T14)  [unwired: 1 in]
                  n314 = Index Array(array=w678, index #2=1 ("index")) -> (element #1=w676:string, element #2=w675:string)  [unwired: 1 in]
                  n315 = property on="Intensity Graph 8" class="IntGraph (strict)"("YScale.NameLbl.Text"=w675) -> ()  [unwired: 2 in, 2 out]
                  n316 = property on="Intensity Graph 7" class="IntGraph (strict)"("YScale.NameLbl.Text"=w676) -> ()  [unwired: 2 in, 2 out]
                  n317 = call "DataVIS_Decimate+Fill_Intensity_Plot.vi"("Log Scale (T)"="Log scale? 5", "fake point value"="fake pt value 4", "Decimate Controls"=w659, "X and Y Arrays to decimate"=w660) -> ("Offset X Low"=w654:dbl, "Decimated X values"=w655:dbl[], "Arr of Y arrays (intensity info)"=w651:dbl[][])  [unwired: 4 in, 1 out]
                  "Intensity Graph 7" <- w651
                  n318 = for {
                    tunnel: w674 -> [w716]
                    tunnel: w694 -> [w715]
                    tunnel: w693 -> [w710] mode=indexing
                    tunnel: w692 -> [w711] mode=indexing
                    tunnel: [w714] -> w691 mode=indexing
                    tunnel: w689 -> [w713]
                    tunnel: [w712] -> w683 mode=indexing
                    tunnel: "X Step 2t" -> [w709]
                    tunnel: "X High 2t" -> [w708]
                    tunnel: "X Low 2t" -> [w707]
                    tunnel: [w704] -> _ mode=indexing
                    n319 = Index Array(array=w713, index (row)=w711, index (col)=w710) -> (element=w712:dbl)
                    n320 = Index Array(array=w716, index (dim 0)=w715, index (dim 1)=w710, index (dim 2)=w711) -> (element=w706:T7)
                    n321 = call <userlib>:"Decimate_VS_X_Value.vi"("XY Graph kind 1"=w706, "X Step"=w709, "X High"=w708, "X Low"=w707) -> ("Interpolated"=w705:cluster{dbl[], dbl[]})  [unwired: 6 in, 1 out]
                    n322 = Unbundle(w705) -> (w704:dbl[], w714:dbl[])
                  }
                  n323 = control-ref of="Intensity Graph 8"() -> (w663:refnum<vi>)
                  n324 = Index Array(array=w683, index #1=0 ("index"), index #2=1 ("index")) -> (element #1=w687:dbl, element #2=w686:dbl)
                  n325 = control-ref of="Intensity Graph 7"() -> (w664:refnum<vi>)
                  n326 = Transpose 2D Array(2D array=w691) -> (transposed array=w690:dbl[][])
                  n327 = Subtract(x=w686, y=w687) -> (x-y=w688:dbl)
                  n328 = case shown="True" "Log scale? 4" {
                    tunnel: w690 -> [w701 w703]
                    tunnel: [w701 w702] -> w681
                    frame False {
                    }
                    frame True {
                      n329 = Logarithm Base 10(1:w703) -> (0:w702:dbl[][])
                    }
                  }
                  "Intensity Graph 8" <- w681
                  n330 = Bundle(w687, w688) -> (w680:cluster{dbl, dbl})  [unwired: 1 in]
                  n331 = property on="Intensity Graph 8" class="IntGraph (strict)"("YScale.Ofst&Mult"=w680) -> ()  [unwired: 2 in, 2 out]
                  n332 = Bundle("Offset X Low"=w654, "X Step 2t"="X Step 2t") -> (w666:cluster{"Offset X Low":dbl, "X Step 2t":dbl})  [unwired: 1 in]
                  n333 = property on="Property Node" class="IntGraph (strict)"(reference=w664, "XScale.Ofst&Mult"=w666) -> ()  [unwired: 1 in, 2 out]
                  n334 = property on="Property Node" class="IntGraph (strict)"(reference=w663, "XScale.Ofst&Mult"=w666) -> ()  [unwired: 1 in, 2 out]
                  n335 = property on="Property Node" class="IntGraph (strict)"(reference=w664) -> ("Cursor.Cursor Plot"=w668:i32)  [unwired: 1 in, 2 out]
                  n336 = property on="Property Node" class="IntGraph (strict)"(reference=w664) -> ("Cursor.Cursor Index"=w667:i32)  [unwired: 1 in, 2 out]
                  n337 = Index Array(array=w651, index (col)=w668) -> (element=w670:dbl[])  [unwired: 1 in]
                  n338 = Index Array(array=w651, index (row)=w667) -> (element=w671:dbl[])  [unwired: 1 in]
                  n339 = Divide(x=w670, y=w669) -> (x/y=w672:dbl[])
                  n340 = Divide(x=w671, y=w669) -> (x/y=w673:dbl[])
                  n341 = Bundle("Decimated X values"=w655, w672) -> (→"X line cut 4":cluster{"Decimated X values":dbl[], dbl[]})  [unwired: 1 in]
                  n342 = Bundle("Vfast"=w665, w673) -> (→"Y line cut 4":cluster{"Vfast":dbl[], dbl[]})  [unwired: 1 in]
                }
                frame "3D" {
                  n343 = for {
                    tunnel: w717 -> [w830] mode=indexing
                    tunnel: [w829] -> w725 mode=indexing
                    tunnel: [w828] -> w729
                    n344 = for {
                      tunnel: w830 -> [w833] mode=indexing
                      tunnel: [w832] -> w829 mode=indexing
                      tunnel: [w831] -> w828
                      n345 = for {
                        tunnel: w833 -> [w840] mode=indexing
                        tunnel: [w842] -> w832 mode=indexing
                        tunnel: [w841] -> w831
                        w835 = u16 0 items=["Mean", "Max", "Min", "Sigma", "Median"] ("Method")
                        n346 = local read "X Step"() -> (w836:dbl)
                        n347 = local read "X Low"() -> (w838:dbl)
                        n348 = local read "X High"() -> (w837:dbl)
                        n349 = local read "fake point value"() -> (w834:dbl)
                        n350 = call <userlib>:"Decimate_VS_X_Value.vi"("fake point value"=w834, "XY Graph kind 1"=w840, "Method"=w835, "X Step"=w836, "X High"=w837, "X Low"=w838) -> ("Interpolated"=w839:cluster{dbl[], dbl[]})  [unwired: 4 in, 1 out]
                        n351 = Unbundle(w839) -> (w841:dbl[], w842:dbl[])
                      }
                    }
                  }
                  n352 = Index Array(array=w735, index #1=0 ("index"), index #2=1 ("index")) -> (element #1=w739:dbl, element #2=w738:dbl)
                  n353 = property on="Intensity Graph 9" class="IntGraph (strict)"() -> ("Cursor.Cursor Index"=w753:i32, "Cursor.Cursor Plot"=w747:i32)  [unwired: 2 in, 2 out]
                  n354 = Index Array(array=w743, index (row)=w741) -> (element=w742:dbl[])  [unwired: 1 in]
                  n355 = Subtract(x=w738, y=w739) -> (x-y=w740:dbl)
                  n356 = Bundle(w739, w740) -> (w724:cluster{dbl, dbl})  [unwired: 1 in]
                  n357 = Index Array(array=w742, index #1=0 ("index"), index #2=1 ("index")) -> (element #1=w723:dbl, element #2=w744:dbl)
                  n358 = property on="Intensity Graph 10" class="IntGraph (strict)"("Cursor.Cursor Plot"=w747) -> ("Cursor.Cursor Index"=w752:i32)  [unwired: 2 in, 2 out]
                  n359 = Subtract(x=w744, y=w723) -> (x-y=w722:dbl)
                  n360 = local read "X scale"() -> (w720:cluster{dbl, "X Step":dbl})
                  n361 = Bundle(w723, w722) -> (w719:cluster{dbl, dbl})  [unwired: 1 in]
                  n362 = Index Array(array=w729, index #1=0 ("index"), index #2=1 ("index")) -> (element #1=w733:dbl, element #2=w732:dbl)
                  n363 = property on="Intensity Graph 9" class="IntGraph (strict)"("XScale.Ofst&Mult"=w719, "YScale.Ofst&Mult"=w720) -> ()  [unwired: 2 in, 2 out]
                  n364 = property on="Transconductance 2" class="IntGraph (strict)"("XScale.Ofst&Mult"=w724, "YScale.Ofst&Mult"=w719) -> ()  [unwired: 2 in, 2 out]
                  n365 = property on="Intensity Graph 10" class="IntGraph (strict)"("XScale.Ofst&Mult"=w724, "YScale.Ofst&Mult"=w720) -> ()  [unwired: 2 in, 2 out]
                  n366 = property on="Intensity Graph 11" class="IntGraph (strict)"("XScale.Ofst&Mult"=w724, "YScale.Ofst&Mult"=w719) -> ()  [unwired: 2 in, 2 out]
                  n367 = Index Array(array=w725, index (dim 0)=0 ("index (vol)"), index (dim 1)=w752) -> (element=→"Intensity Graph 9":dbl[][])  [unwired: 2 in]
                  n368 = Index Array(array=w725, index (dim 0)=0 ("disabled index (page) 2"), index (dim 2)=w753) -> (element=→"Intensity Graph 10":dbl[][])  [unwired: 2 in]
                  n369 = Subtract(x=w732, y=w733) -> (x-y=w734:dbl)
                  n370 = Bundle(w733, w734) -> ()  [unwired: 1 in, 1 out]
                  n371 = Index Array(array=w725, index (dim 0)=0 ("disabled index (row) 2"), index (dim 3)=w747) -> (element=w728:dbl[][])  [unwired: 2 in]
                  "Intensity Graph 11" <- w728
                  n372 = call "transcond_intensity_v2.vi"("derivative bin size"="derivative bin size 2", "Conductance"=w728) -> ("Transconductance"=w726:dbl[][])  [unwired: 9 in]
                  "Transconductance 2" <- w726
                  n373 = case shown="True" "calc alpha?" {
                    tunnel: w726 -> [_ w770]
                    tunnel: w725 -> [_ w769]
                    tunnel: w724 -> [_ w768]
                    tunnel: w720 -> [_ w767]
                    tunnel: w719 -> [_ w766]
                    frame False {
                    }
                    frame True {
                      # "all of this should go in a separate state. or otherwise only run on demand"
                      n374 = Unbundle(w768) -> (w759:dbl, w758:dbl)
                      n375 = for {
                        tunnel: w770 -> [w827] mode=indexing
                        tunnel: [w813] -> w756 mode=indexing
                        tunnel: w759 -> [w824]
                        tunnel: w758 -> [w823]
                        shift-right: [w820] -> w762
                        shift-left: dbl[] [] -> [w818]
                        tunnel: [w817] -> w755 mode=indexing
                        tunnel: w766 -> [w814]
                        tunnel: [w804] -> w761 mode=indexing
                        i -> [w822]
                        w807 = 1 ("index")
                        w808 = 0 ("index")
                        n376 = Unbundle(w814) -> (w811:dbl, w812:dbl)
                        n377 = Multiply(x=w823, y=w822) -> (x*y=w821:dbl)
                        n378 = Add(x=w824, y=w821) -> (x+y=w819:dbl)
                        n379 = call <vilib>:"Peak Detector.vi"("width"="width", "threshold"="threshold", "X"=w827) -> ("Locations"=w810:dbl[])  [unwired: 4 in, 4 out]
                        n380 = Multiply(x=w810, y=w812) -> (x*y=w815:dbl[])
                        n381 = Build Array (concatenate)(w818, w819) -> (w820:dbl[])
                        n382 = Add(x=w815, y=w811) -> (x+y=w809:dbl[])
                        n383 = Index Array(array=w810, index #1=w808, index #2=w807) -> (element #1=w817:dbl, element #2=w816:dbl)
                        n384 = Index Array(array=w809, index #1=w808, index #2=w807) -> (element #1=w805:dbl, element #2=w806:dbl)
                        n385 = Subtract(x=w816, y=w817) -> (x-y=w813:dbl)
                        n386 = Subtract(x=w806, y=w805) -> (x-y=w804:dbl)
                      }
                      "vertical peak diff" <- w756
                      n387 = for {
                        tunnel: w769 -> [w803]
                        tunnel: w756 -> [w786] mode=indexing
                        tunnel: [w784] -> _ mode=indexing
                        tunnel: w755 -> [w790] mode=indexing
                        tunnel: w767 -> [w781]
                        tunnel: [w775] -> w754 mode=indexing
                        i -> [w801]
                        n388 = local read "derivative bin size"() -> (w800:dbl)
                        n389 = Unbundle(w781) -> (w773:dbl, "X Step"=w774:dbl)
                        n390 = Index Array(array=w803, index (dim 0)=0 ("index (vol)"), index (dim 1)=w801) -> (element=w794:dbl[][])  [unwired: 2 in]
                        n391 = Divide(x=w786, y=2.0) -> (x/y=w789:dbl)
                        n392 = Transpose 2D Array(2D array=w794) -> (transposed array=w793:dbl[][])
                        n393 = Add(x=w790, y=w789) -> (x+y=w788:dbl)
                        n394 = call "transcond_intensity_v2.vi"("derivative bin size"=w800, "Conductance"=w793) -> ("Transconductance"=w792:dbl[][])  [unwired: 9 in]
                        n395 = Transpose 2D Array(2D array=w792) -> (transposed array=w791:dbl[][])
                        "Intensity Graph 12" <- w791
                        n396 = Index Array(array=w791, index (row)=w788) -> (element=w787:dbl[])  [unwired: 1 in]
                        n397 = call <vilib>:"Peak Detector.vi"("peaks/valleys"=enum32{"Peaks", "Valleys"}."Peaks", "width"="width 2", "threshold"="threshold 2", "X"=w787) -> ("Locations"=w779:dbl[])  [unwired: 3 in, 4 out]
                        n398 = Multiply(x=w779, y=w774) -> (x*y=w780:dbl[])
                        n399 = Index Array(array=w779, index #1=0 ("index"), index #2=1 ("index")) -> (element #1=w783:dbl, element #2=w782:dbl)
                        n400 = Add(x=w780, y=w773) -> (x+y=w778:dbl[])
                        n401 = Subtract(x=w782, y=w783) -> (x-y=w784:dbl)
                        n402 = Index Array(array=w778, index #1=0 ("index"), index #2=1 ("index")) -> (element #1=w771:dbl, element #2=w772:dbl)
                        n403 = Subtract(x=w772, y=w771) -> (x-y=w775:dbl)
                      }
                      "Array 2" <- w754
                      n404 = Bundle(w761, w754) -> (→"Vsd vs Vsg":cluster{dbl[], dbl[]})  [unwired: 1 in]
                      n405 = Bundle(w762, w754) -> (w763:cluster{dbl[], dbl[]})  [unwired: 1 in]
                      n406 = Bundle(w762, w761) -> (w765:cluster{dbl[], dbl[]})  [unwired: 1 in]
                      n407 = Build Array(w763, w765) -> (→"Y line cut 9":cluster{dbl[], dbl[]}[])
                    }
                  }
                }
                frame "Whatever" {
                  # "if I want dV/dI 2T:"
                  n408 = for {
                    tunnel: w843 -> [_] mode=indexing
                  }
                }
              }
              n409 = in-place-dvr #5(w219) -> (w203:refnum<data-value>)  [unwired: 1 out]
              n410 = in-place-dvr #6(w220) -> (w202:refnum<data-value>)  [unwired: 1 out]
              n411 = in-place-dvr #7(w221) -> (w212:refnum<data-value>)  [unwired: 1 out]
              n412 = in-place-dvr #8(w222) -> (w206:refnum<data-value>)  [unwired: 1 out]
              n413 = in-place-dvr #9(w224) -> (w205:refnum<data-value>)  [unwired: 1 out]
              n414 = in-place-dvr #10(w223) -> (w204:refnum<data-value>)  [unwired: 1 out]
            }
          }
          frame 4 {
          }
        }
      }
      n415 = Delete Data Value Reference(data value reference=w6) -> ()  [unwired: 1 in, 2 out]
      n416 = Delete Data Value Reference(data value reference=w5) -> ()  [unwired: 1 in, 2 out]
      n417 = Delete Data Value Reference(data value reference=w10) -> ()  [unwired: 1 in, 2 out]
      n418 = Delete Data Value Reference(data value reference=w9) -> ()  [unwired: 1 in, 2 out]
      n419 = Delete Data Value Reference(data value reference=w8) -> ()  [unwired: 1 in, 2 out]
      n420 = Delete Data Value Reference(data value reference=w7) -> ()  [unwired: 1 in, 2 out]
    }
    frame True {
      # "Generate"
      n421 = for {
        N: "# of fields/Temperatures" -> [_]
        tunnel: [w909] -> w873 mode=indexing
        tunnel: [w904] -> w859
        tunnel: [w903] -> w858
        tunnel: [w902] -> w862 mode=indexing
        tunnel: [w884] -> w857 mode=indexing
        tunnel: "# of fields/Temperatures" -> [_]
        tunnel: "# of fields/Temperatures" -> [w892]
        tunnel: [w883] -> w860
        tunnel: ["Scan names"] -> w856
        i -> [w908]
        n422 = Multiply(x="Field Period", y=w908) -> (x*y=w905:i32)
        n423 = Cluster To Array(cluster="IV setup") -> (array=w901:i32[])
        n424 = Bundle By Name(cluster="IV setup", "B/T offset"=w905) -> (w897:T2)
        n425 = call "Data retrieve engine_SE.vi"("File or Folder Path"="File or Folder Path", "Scan names"="Scan names", "IV setup"=w897, "index"="index 2", "Portion of data"="Portion of data", "Decimate point"="Decimate point", "Extract paramaters from comments?"="Extract parameters from comments?") -> ("Comments"=w878:string, "IV"=w909:cluster{dbl[], dbl[]}[][], "IV-2T"=w902:cluster{dbl[], dbl[]}[][], "Vfast"=w904:dbl[][], "Vslow"=w903:dbl[], "N"=w906:cluster{"N1":dbl, "N2":dbl, "N3":dbl, "N4":dbl}, "Vslowest"=w887:dbl)  [unwired: 2 in]
        n426 = Unbundle By Name(w906) -> ("N1"=w886:dbl)
        n427 = for {
          tunnel: w901 -> [w918] mode=indexing
          shift-right: [w915] -> w894
          shift-left: "" -> [w914]
          n428 = Format Into String(w918) -> (resulting string=w917:string)  [unwired: 3 in, 1 out]
          n429 = Concatenate Strings(w914, "/" ("string"), w917) -> (w915:string)
        }
        n430 = for {
          tunnel: "Scan names" -> [w911] mode=indexing
          shift-right: [w913] -> w880
          shift-left: "" -> [w912]
          n431 = Concatenate Strings(w912, "\n" ("string"), w911) -> (w913:string)
        }
        n432 = Select(t=w887, s="T/B     third axis", f=w886) -> (s? t:f=w884:dbl)
        n433 = Format Into String(initial string="Additional comments", "      #Vslow/#Vfast/# of IV curves/BT offset/#discarded IV curves/Manual offset:\n" ("string"), w894, "   \n#of fields:" ("string"), w892, "   \nField period" ("string"), "Field Period", "\nDecimate point", "Decimate point", "\nScan names", w880, "\n" ("input 11"), w878) -> (resulting string=w883:string)  [unwired: 2 in, 1 out]
      }
      n434 = Bundle("IV"=w873, "IV-2T"=w862, "Vfast"=w859, "Vslow"=w858, w857, w860, "Scan names"=w856) -> (w863:T15)  [unwired: 1 in]
      n435 = Build Path(base path="Processed data folder", name or relative path="IV file name") -> (appended path=w864:path)
      n436 = Open/Create/Replace File(file path (use dialog)=w864, operation (0:open)=T4."replace or create", access (0:read/write)=enum16{"read/write", "read-only", "write-only"}."read/write") -> (refnum out=w868:refnum<file>, error out=w869:errorcluster)  [unwired: 3 in, 1 out]
      n437 = Write to Binary File(file (use dialog)=w868, data=w863, error in=w869) -> (refnum out=w872:refnum<file>, error out=w871:errorcluster)  [unwired: 3 in, 1 out]
      n438 = Close File(refnum=w872, error in=w871) -> (error out=w870:errorcluster)  [unwired: 1 out]
      n439 = call <vilib>:"Simple Error Handler.vi"("error in (no error)"=w870) -> ()  [unwired: 4 in, 5 out]
    }
  }
  n440 = Request Deallocation(w1) -> ()
